vi "Crazy.vi"() -> ()   [LabVIEW 2014]
uses:
  <vilib>/Utility/inputDevices.llb/keyboardAcquire.vi
  <vilib>/Utility/inputDevices.llb/closeKeyboard.vi
panel:
  out "Å]YÄ²2":i32
  out "Å]XÄ²2":i32
  out "Å]Vy2":i32
  out "Å]Vx2":i32
  out "魔王2":bool
  out "Å]YÄ²1":i32
  out "Å]XÄ²1":i32
  out "Å]Vy1":i32
  out "Å]Vx1":i32
  out "魔王1":bool
  out "Vx 2":i32
  out "x觸及位置 2":i32
  out "X障礙 2":bool
  out "y觸及位置 2":i32
  out "Vy 2":i32
  out "Y障礙 2":bool
  out "Å]YÄ²":i32
  out "Å]XÄ²":i32
  out "Å]Vy":i64
  out "Å]Vx":i32
  out "魔王":bool
  out "終點":bool
  out "遊玩時間":i32
  out "X障礙":bool
  out "Y位置 2":i32
  out "x位置 2":i32
  out "X":dbl
  out "Y":dbl
  out "小精靈":bool
  out "x位置":i32
  out "Y位置":i32
  out "Y障礙":bool
  out "x觸及位置":i32
  out "y觸及位置":i32
  out "x-y":u32
  out "Vy":i32
  out "Vx":i32
  # "小精靈"
  # "500"
  # "障礙"
  # "400"
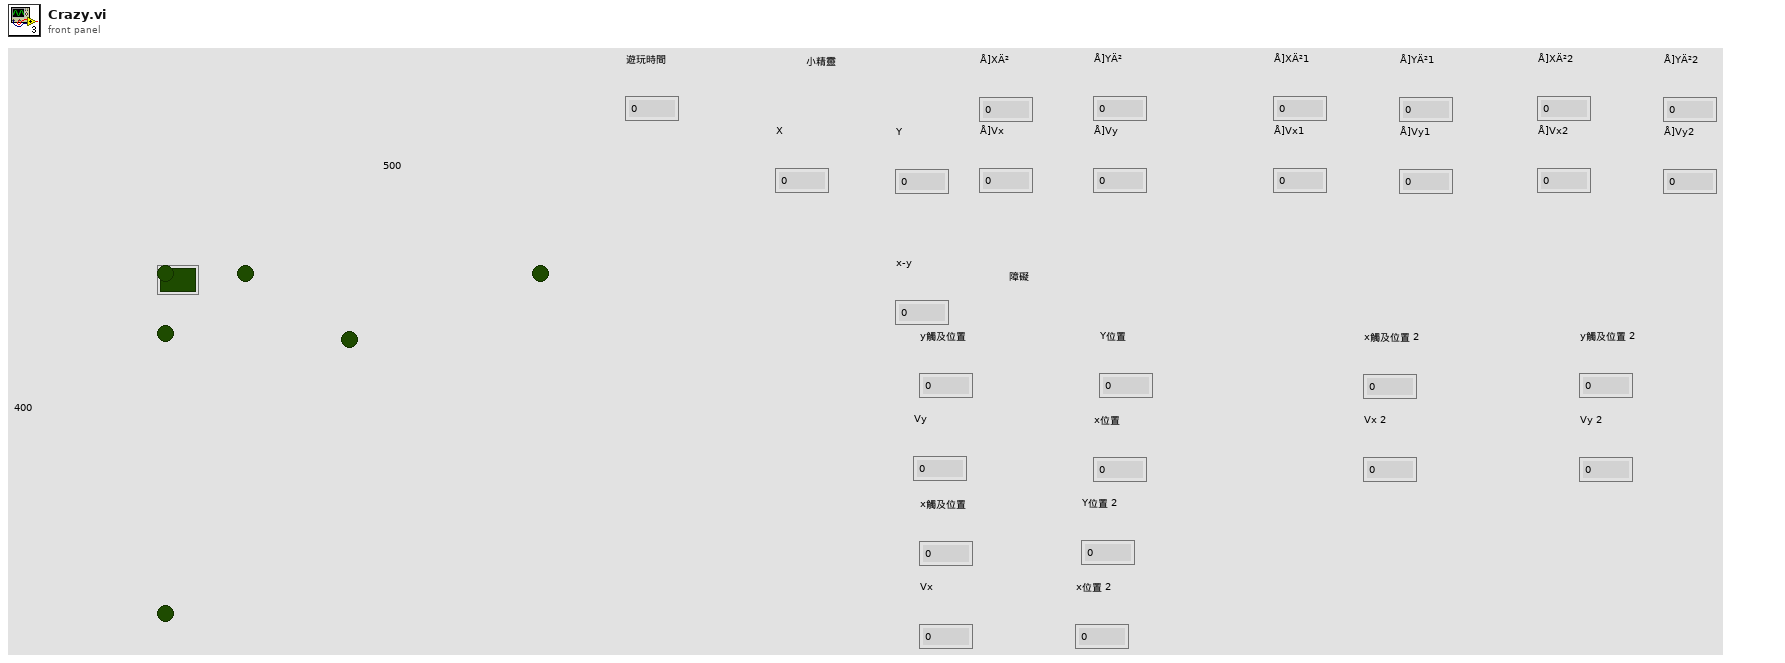
[diagram p1: front panel]
types:
  T1 = enum16{"0", "1", "2", "3", "4", "5", "6", "7", "8", "9", "A", "B", "C", "D", "E", "F", "G", "H", "I", "J", "K", "L", "M", "N", "O", "P", "Q", "R", "S", "T", "U", "V", "W", "X", "Y", "Z", "F1", "F2", "F3", "F4", "F5", "F6", "F7", "F8", "F9", "F10", "F11", "F12", "F13", "F14", "F15", "ADD", "BACK", "BACKSLASH", "CAPITAL", "COMMA", "DECIMAL", "DELETE", "DIVIDE", "DOWN", "END", "EQUALS", "ESCAPE", "GRAVE (`)", "HOME", "INSERT", "LBRACKET", "LCONTROL", "LEFT", "L ALT", "LSHIFT", "LWIN", "MINUS", "MULTIPLY", "NEXT", "NUMLOCK", "NUMPAD_0", "NUMPAD_1", "NUMPAD_2", "NUMPAD_3", "NUMPAD_4", "NUMPAD_5", "NUMPAD_6", "NUMPAD_7", "NUMPAD_8", "NUMPAD_9", "PAUSE", "PERIOD", "PRIOR (PG UP)", "RBRACKET", "RCONTROL", "RETURN", "RIGHT", "R ALT", "RSHIFT", "RWIN", "SCROLL", "SEMICOLON", "SLASH", "SPACE", "SUBTRACT", "TAB", "UP", "ENTER (num pad)", "' (quote)"}[]
  T2 = cluster{"keys pressed[0]":enum16{"0", "1", "2", "3", "4", "5", "6", "7", "8", "9", "A", "B", "C", "D", "E", "F", "G", "H", "I", "J", "K", "L", "M", "N", "O", "P", "Q", "R", "S", "T", "U", "V", "W", "X", "Y", "Z", "F1", "F2", "F3", "F4", "F5", "F6", "F7", "F8", "F9", "F10", "F11", "F12", "F13", "F14", "F15", "ADD", "BACK", "BACKSLASH", "CAPITAL", "COMMA", "DECIMAL", "DELETE", "DIVIDE", "DOWN", "END", "EQUALS", "ESCAPE", "GRAVE (`)", "HOME", "INSERT", "LBRACKET", "LCONTROL", "LEFT", "L ALT", "LSHIFT", "LWIN", "MINUS", "MULTIPLY", "NEXT", "NUMLOCK", "NUMPAD_0", "NUMPAD_1", "NUMPAD_2", "NUMPAD_3", "NUMPAD_4", "NUMPAD_5", "NUMPAD_6", "NUMPAD_7", "NUMPAD_8", "NUMPAD_9", "PAUSE", "PERIOD", "PRIOR (PG UP)", "RBRACKET", "RCONTROL", "RETURN", "RIGHT", "R ALT", "RSHIFT", "RWIN", "SCROLL", "SEMICOLON", "SLASH", "SPACE", "SUBTRACT", "TAB", "UP", "ENTER (num pad)", "' (quote)"}, "keys pressed[1]":enum16{"0", "1", "2", "3", "4", "5", "6", "7", "8", "9", "A", "B", "C", "D", "E", "F", "G", "H", "I", "J", "K", "L", "M", "N", "O", "P", "Q", "R", "S", "T", "U", "V", "W", "X", "Y", "Z", "F1", "F2", "F3", "F4", "F5", "F6", "F7", "F8", "F9", "F10", "F11", "F12", "F13", "F14", "F15", "ADD", "BACK", "BACKSLASH", "CAPITAL", "COMMA", "DECIMAL", "DELETE", "DIVIDE", "DOWN", "END", "EQUALS", "ESCAPE", "GRAVE (`)", "HOME", "INSERT", "LBRACKET", "LCONTROL", "LEFT", "L ALT", "LSHIFT", "LWIN", "MINUS", "MULTIPLY", "NEXT", "NUMLOCK", "NUMPAD_0", "NUMPAD_1", "NUMPAD_2", "NUMPAD_3", "NUMPAD_4", "NUMPAD_5", "NUMPAD_6", "NUMPAD_7", "NUMPAD_8", "NUMPAD_9", "PAUSE", "PERIOD", "PRIOR (PG UP)", "RBRACKET", "RCONTROL", "RETURN", "RIGHT", "R ALT", "RSHIFT", "RWIN", "SCROLL", "SEMICOLON", "SLASH", "SPACE", "SUBTRACT", "TAB", "UP", "ENTER (num pad)", "' (quote)"}, "keys pressed[2]":enum16{"0", "1", "2", "3", "4", "5", "6", "7", "8", "9", "A", "B", "C", "D", "E", "F", "G", "H", "I", "J", "K", "L", "M", "N", "O", "P", "Q", "R", "S", "T", "U", "V", "W", "X", "Y", "Z", "F1", "F2", "F3", "F4", "F5", "F6", "F7", "F8", "F9", "F10", "F11", "F12", "F13", "F14", "F15", "ADD", "BACK", "BACKSLASH", "CAPITAL", "COMMA", "DECIMAL", "DELETE", "DIVIDE", "DOWN", "END", "EQUALS", "ESCAPE", "GRAVE (`)", "HOME", "INSERT", "LBRACKET", "LCONTROL", "LEFT", "L ALT", "LSHIFT", "LWIN", "MINUS", "MULTIPLY", "NEXT", "NUMLOCK", "NUMPAD_0", "NUMPAD_1", "NUMPAD_2", "NUMPAD_3", "NUMPAD_4", "NUMPAD_5", "NUMPAD_6", "NUMPAD_7", "NUMPAD_8", "NUMPAD_9", "PAUSE", "PERIOD", "PRIOR (PG UP)", "RBRACKET", "RCONTROL", "RETURN", "RIGHT", "R ALT", "RSHIFT", "RWIN", "SCROLL", "SEMICOLON", "SLASH", "SPACE", "SUBTRACT", "TAB", "UP", "ENTER (num pad)", "' (quote)"}, "keys pressed[3]":enum16{"0", "1", "2", "3", "4", "5", "6", "7", "8", "9", "A", "B", "C", "D", "E", "F", "G", "H", "I", "J", "K", "L", "M", "N", "O", "P", "Q", "R", "S", "T", "U", "V", "W", "X", "Y", "Z", "F1", "F2", "F3", "F4", "F5", "F6", "F7", "F8", "F9", "F10", "F11", "F12", "F13", "F14", "F15", "ADD", "BACK", "BACKSLASH", "CAPITAL", "COMMA", "DECIMAL", "DELETE", "DIVIDE", "DOWN", "END", "EQUALS", "ESCAPE", "GRAVE (`)", "HOME", "INSERT", "LBRACKET", "LCONTROL", "LEFT", "L ALT", "LSHIFT", "LWIN", "MINUS", "MULTIPLY", "NEXT", "NUMLOCK", "NUMPAD_0", "NUMPAD_1", "NUMPAD_2", "NUMPAD_3", "NUMPAD_4", "NUMPAD_5", "NUMPAD_6", "NUMPAD_7", "NUMPAD_8", "NUMPAD_9", "PAUSE", "PERIOD", "PRIOR (PG UP)", "RBRACKET", "RCONTROL", "RETURN", "RIGHT", "R ALT", "RSHIFT", "RWIN", "SCROLL", "SEMICOLON", "SLASH", "SPACE", "SUBTRACT", "TAB", "UP", "ENTER (num pad)", "' (quote)"}, "keys pressed[4]":enum16{"0", "1", "2", "3", "4", "5", "6", "7", "8", "9", "A", "B", "C", "D", "E", "F", "G", "H", "I", "J", "K", "L", "M", "N", "O", "P", "Q", "R", "S", "T", "U", "V", "W", "X", "Y", "Z", "F1", "F2", "F3", "F4", "F5", "F6", "F7", "F8", "F9", "F10", "F11", "F12", "F13", "F14", "F15", "ADD", "BACK", "BACKSLASH", "CAPITAL", "COMMA", "DECIMAL", "DELETE", "DIVIDE", "DOWN", "END", "EQUALS", "ESCAPE", "GRAVE (`)", "HOME", "INSERT", "LBRACKET", "LCONTROL", "LEFT", "L ALT", "LSHIFT", "LWIN", "MINUS", "MULTIPLY", "NEXT", "NUMLOCK", "NUMPAD_0", "NUMPAD_1", "NUMPAD_2", "NUMPAD_3", "NUMPAD_4", "NUMPAD_5", "NUMPAD_6", "NUMPAD_7", "NUMPAD_8", "NUMPAD_9", "PAUSE", "PERIOD", "PRIOR (PG UP)", "RBRACKET", "RCONTROL", "RETURN", "RIGHT", "R ALT", "RSHIFT", "RWIN", "SCROLL", "SEMICOLON", "SLASH", "SPACE", "SUBTRACT", "TAB", "UP", "ENTER (num pad)", "' (quote)"}, "keys pressed[5]":enum16{"0", "1", "2", "3", "4", "5", "6", "7", "8", "9", "A", "B", "C", "D", "E", "F", "G", "H", "I", "J", "K", "L", "M", "N", "O", "P", "Q", "R", "S", "T", "U", "V", "W", "X", "Y", "Z", "F1", "F2", "F3", "F4", "F5", "F6", "F7", "F8", "F9", "F10", "F11", "F12", "F13", "F14", "F15", "ADD", "BACK", "BACKSLASH", "CAPITAL", "COMMA", "DECIMAL", "DELETE", "DIVIDE", "DOWN", "END", "EQUALS", "ESCAPE", "GRAVE (`)", "HOME", "INSERT", "LBRACKET", "LCONTROL", "LEFT", "L ALT", "LSHIFT", "LWIN", "MINUS", "MULTIPLY", "NEXT", "NUMLOCK", "NUMPAD_0", "NUMPAD_1", "NUMPAD_2", "NUMPAD_3", "NUMPAD_4", "NUMPAD_5", "NUMPAD_6", "NUMPAD_7", "NUMPAD_8", "NUMPAD_9", "PAUSE", "PERIOD", "PRIOR (PG UP)", "RBRACKET", "RCONTROL", "RETURN", "RIGHT", "R ALT", "RSHIFT", "RWIN", "SCROLL", "SEMICOLON", "SLASH", "SPACE", "SUBTRACT", "TAB", "UP", "ENTER (num pad)", "' (quote)"}, "keys pressed[6]":enum16{"0", "1", "2", "3", "4", "5", "6", "7", "8", "9", "A", "B", "C", "D", "E", "F", "G", "H", "I", "J", "K", "L", "M", "N", "O", "P", "Q", "R", "S", "T", "U", "V", "W", "X", "Y", "Z", "F1", "F2", "F3", "F4", "F5", "F6", "F7", "F8", "F9", "F10", "F11", "F12", "F13", "F14", "F15", "ADD", "BACK", "BACKSLASH", "CAPITAL", "COMMA", "DECIMAL", "DELETE", "DIVIDE", "DOWN", "END", "EQUALS", "ESCAPE", "GRAVE (`)", "HOME", "INSERT", "LBRACKET", "LCONTROL", "LEFT", "L ALT", "LSHIFT", "LWIN", "MINUS", "MULTIPLY", "NEXT", "NUMLOCK", "NUMPAD_0", "NUMPAD_1", "NUMPAD_2", "NUMPAD_3", "NUMPAD_4", "NUMPAD_5", "NUMPAD_6", "NUMPAD_7", "NUMPAD_8", "NUMPAD_9", "PAUSE", "PERIOD", "PRIOR (PG UP)", "RBRACKET", "RCONTROL", "RETURN", "RIGHT", "R ALT", "RSHIFT", "RWIN", "SCROLL", "SEMICOLON", "SLASH", "SPACE", "SUBTRACT", "TAB", "UP", "ENTER (num pad)", "' (quote)"}, "keys pressed[7]":enum16{"0", "1", "2", "3", "4", "5", "6", "7", "8", "9", "A", "B", "C", "D", "E", "F", "G", "H", "I", "J", "K", "L", "M", "N", "O", "P", "Q", "R", "S", "T", "U", "V", "W", "X", "Y", "Z", "F1", "F2", "F3", "F4", "F5", "F6", "F7", "F8", "F9", "F10", "F11", "F12", "F13", "F14", "F15", "ADD", "BACK", "BACKSLASH", "CAPITAL", "COMMA", "DECIMAL", "DELETE", "DIVIDE", "DOWN", "END", "EQUALS", "ESCAPE", "GRAVE (`)", "HOME", "INSERT", "LBRACKET", "LCONTROL", "LEFT", "L ALT", "LSHIFT", "LWIN", "MINUS", "MULTIPLY", "NEXT", "NUMLOCK", "NUMPAD_0", "NUMPAD_1", "NUMPAD_2", "NUMPAD_3", "NUMPAD_4", "NUMPAD_5", "NUMPAD_6", "NUMPAD_7", "NUMPAD_8", "NUMPAD_9", "PAUSE", "PERIOD", "PRIOR (PG UP)", "RBRACKET", "RCONTROL", "RETURN", "RIGHT", "R ALT", "RSHIFT", "RWIN", "SCROLL", "SEMICOLON", "SLASH", "SPACE", "SUBTRACT", "TAB", "UP", "ENTER (num pad)", "' (quote)"}, "keys pressed[8]":enum16{"0", "1", "2", "3", "4", "5", "6", "7", "8", "9", "A", "B", "C", "D", "E", "F", "G", "H", "I", "J", "K", "L", "M", "N", "O", "P", "Q", "R", "S", "T", "U", "V", "W", "X", "Y", "Z", "F1", "F2", "F3", "F4", "F5", "F6", "F7", "F8", "F9", "F10", "F11", "F12", "F13", "F14", "F15", "ADD", "BACK", "BACKSLASH", "CAPITAL", "COMMA", "DECIMAL", "DELETE", "DIVIDE", "DOWN", "END", "EQUALS", "ESCAPE", "GRAVE (`)", "HOME", "INSERT", "LBRACKET", "LCONTROL", "LEFT", "L ALT", "LSHIFT", "LWIN", "MINUS", "MULTIPLY", "NEXT", "NUMLOCK", "NUMPAD_0", "NUMPAD_1", "NUMPAD_2", "NUMPAD_3", "NUMPAD_4", "NUMPAD_5", "NUMPAD_6", "NUMPAD_7", "NUMPAD_8", "NUMPAD_9", "PAUSE", "PERIOD", "PRIOR (PG UP)", "RBRACKET", "RCONTROL", "RETURN", "RIGHT", "R ALT", "RSHIFT", "RWIN", "SCROLL", "SEMICOLON", "SLASH", "SPACE", "SUBTRACT", "TAB", "UP", "ENTER (num pad)", "' (quote)"}}
  T3 = enum16{"0", "1", "2", "3", "4", "5", "6", "7", "8", "9", "A", "B", "C", "D", "E", "F", "G", "H", "I", "J", "K", "L", "M", "N", "O", "P", "Q", "R", "S", "T", "U", "V", "W", "X", "Y", "Z", "F1", "F2", "F3", "F4", "F5", "F6", "F7", "F8", "F9", "F10", "F11", "F12", "F13", "F14", "F15", "ADD", "BACK", "BACKSLASH", "CAPITAL", "COMMA", "DECIMAL", "DELETE", "DIVIDE", "DOWN", "END", "EQUALS", "ESCAPE", "GRAVE (`)", "HOME", "INSERT", "LBRACKET", "LCONTROL", "LEFT", "L ALT", "LSHIFT", "LWIN", "MINUS", "MULTIPLY", "NEXT", "NUMLOCK", "NUMPAD_0", "NUMPAD_1", "NUMPAD_2", "NUMPAD_3", "NUMPAD_4", "NUMPAD_5", "NUMPAD_6", "NUMPAD_7", "NUMPAD_8", "NUMPAD_9", "PAUSE", "PERIOD", "PRIOR (PG UP)", "RBRACKET", "RCONTROL", "RETURN", "RIGHT", "R ALT", "RSHIFT", "RWIN", "SCROLL", "SEMICOLON", "SLASH", "SPACE", "SUBTRACT", "TAB", "UP", "ENTER (num pad)", "' (quote)"}
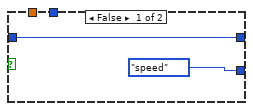
[diagram p3: hidden frame]
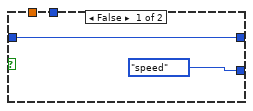
[diagram p5: hidden frame]
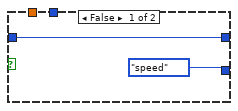
[diagram p7: hidden frame]
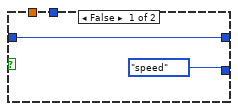
[diagram p9: hidden frame]
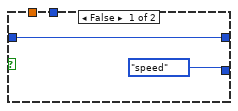
[diagram p11: hidden frame]
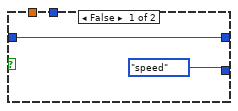
[diagram p17: hidden frame]
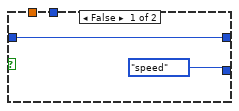
[diagram p19: hidden frame]
diagram:
  n1 = flat-sequence {
    tunnel: [w107] -> w32
    tunnel: [w106] -> w30
    tunnel: [w99] -> w18
    tunnel: [w98] -> w17
    tunnel: [w91] -> w5
    tunnel: [w589] -> w33
    tunnel: w32 -> [w589]
    tunnel: [w588] -> w31
    tunnel: w30 -> [w588]
    tunnel: w18 -> [w567]
    tunnel: w17 -> [w568]
    tunnel: [w568] -> w16
    tunnel: [w567] -> w15
    tunnel: [w566] -> w6
    tunnel: w5 -> [w566]
    tunnel: w33 -> [w633]
    tunnel: w31 -> [w632]
    tunnel: [w623] -> w27
    tunnel: [w622] -> w25
    tunnel: [w621] -> w23
    tunnel: [w620] -> w21
    tunnel: [w619] -> w19
    tunnel: w16 -> [w612]
    tunnel: w15 -> [w611]
    tunnel: [w610] -> w14
    tunnel: [w609] -> w13
    tunnel: [w608] -> w10
    tunnel: [w607] -> w9
    tunnel: w6 -> [w606]
    tunnel: [w605] -> w3
    tunnel: [w598] -> w1
    tunnel: [w1256] -> w28
    tunnel: w27 -> [w1256]
    tunnel: [w1255] -> w26
    tunnel: w25 -> [w1255]
    tunnel: [w1254] -> w24
    tunnel: w23 -> [w1254]
    tunnel: [w1253] -> w22
    tunnel: w21 -> [w1253]
    tunnel: [w1252] -> w20
    tunnel: w19 -> [w1252]
    tunnel: w14 -> [w1237]
    tunnel: w13 -> [w1236]
    tunnel: [w1237] -> w12
    tunnel: [w1236] -> w11
    tunnel: w10 -> [w1235]
    tunnel: w9 -> [w1234]
    tunnel: [w1235] -> w8
    tunnel: [w1234] -> w7
    tunnel: [w1225] -> w4
    tunnel: w3 -> [w1225]
    tunnel: [w1224] -> w2
    tunnel: w1 -> [w1224]
    tunnel: w28 -> [w1300]
    tunnel: w26 -> [w1299]
    tunnel: w24 -> [w1298]
    tunnel: w22 -> [w1297]
    tunnel: w20 -> [w1296]
    tunnel: w12 -> [w1278]
    tunnel: w11 -> [w1277]
    tunnel: w8 -> [w1276]
    tunnel: w7 -> [w1275]
    tunnel: w4 -> [w1268]
    tunnel: w2 -> [w1267]
    frame #0 {
      w38 = 0 ("Å]XÄ²1")
      # "下:小精靈控制"
      # "上:障礙控制"
      n2 = Random Number (0-1)() -> (number: 0 to 1=w80:dbl)
      n3 = Random Number (0-1)() -> (number: 0 to 1=w47:dbl)
      n4 = Random Number (0-1)() -> (number: 0 to 1=w85:dbl)
      n5 = Random Number (0-1)() -> (number: 0 to 1=w41:dbl)
      n6 = Multiply(x=200.0, y=w80) -> (x*y=w78:dbl)
      n7 = Random Number (0-1)() -> (number: 0 to 1=w54:dbl)
      n8 = property on="Y障礙 2" class="Bool (strict)"("Left"=300 ("Position:Left"), "Top"=1 ("Position:Top")) -> ()  [unwired: 2 in, 2 out]
      n9 = Random Number (0-1)() -> (number: 0 to 1=w62:dbl)
      n10 = property on="Y障礙" class="Bool (strict)"("Left"=200 ("Position:Left"), "Top"=1 ("Position:Top")) -> ()  [unwired: 2 in, 2 out]
      n11 = property on="魔王" class="Bool (strict)"("Left"=-500 ("Position:Left"), "Top"=0 ("Position:Top")) -> ()  [unwired: 2 in, 2 out]
      n12 = Add(x=100.0 ("Vy"), y=w78) -> (x+y=→"Vy":dbl)
      n13 = Multiply(x=200.0, y=w54) -> (x*y=w52:dbl)
      n14 = Multiply(x=200.0, y=w47) -> (x*y=w45:dbl)
      n15 = Add(x=300.0 ("y"), y=w45) -> (x+y=→"Å]Vx1":dbl)
      n16 = Multiply(x=200.0, y=w85) -> (x*y=w83:dbl)
      n17 = Add(x=100.0 ("y"), y=w83) -> (x+y=→"Vx":dbl)
      n18 = Multiply(x=200.0, y=w41) -> (x*y=w43:dbl)
      n19 = Add(x=300.0 ("y"), y=w43) -> (x+y=→"Å]Vy1":dbl)
      n20 = Add(x=100.0 ("Vy"), y=w52) -> (x+y=→"Vy 2":dbl)
      n21 = Multiply(x=200.0, y=w62) -> (x*y=w60:dbl)
      n22 = Add(x=100.0 ("y"), y=w60) -> (x+y=→"Vx 2":dbl)
      n23 = property on="小精靈" class="Bool (strict)"("Left"=0 ("Position:Left"), "Top"=100 ("Position:Top")) -> ()  [unwired: 2 in, 2 out]
      n24 = property on="終點" class="Bool (strict)"("Left"=477 ("Position:Left"), "Top"=374 ("Position:Top")) -> ()  [unwired: 2 in, 2 out]
      n25 = property on="X障礙" class="Bool (strict)"("Left"=1 ("Position:Left"), "Top"=200 ("Position:Top")) -> ()  [unwired: 2 in, 2 out]
      n26 = property on="魔王1" class="Bool (strict)"("Left"=-500 ("Position:Left"), "Top"=0 ("Position:Top")) -> ()  [unwired: 2 in, 2 out]
      n27 = property on="魔王2" class="Bool (strict)"("Left"=-500 ("Position:Left"), "Top"=5 ("Position:Top")) -> ()  [unwired: 2 in, 2 out]
      n28 = property on="X障礙 2" class="Bool (strict)"("Left"=1 ("Position:Left"), "Top"=270 ("Position:Top")) -> ()  [unwired: 2 in, 2 out]
      "y觸及位置" <- 0.0 ("x*y")
      "x觸及位置" <- 0.0 ("x*y")
      "小精靈" <- TRUE
      "X" <- 0.0 ("Numeric")
      "Y" <- 100.0 ("Y")
      "遊玩時間" <- 0 ("Numeric")
      "x觸及位置 2" <- 0.0 ("x*y")
      "y觸及位置 2" <- 0.0 ("x*y")
      "Å]XÄ²1" <- w38
      "Å]YÄ²1" <- w38
    }
    frame #1 {
      w92 = 0 ("Top")
      w95 = 0 ("Top")
      w102 = 0 ("Left")
      w103 = 0 ("Left")
      w108 = 0
      w109 = 0
      n29 = call <vilib>:"Intialize Keyboard.vi"() -> ("error out"=w113:errorcluster, "device ID"=w115:refnum<k1>)  [unwired: 10 in]
      n30 = Tick Count (ms)() -> (millisecond timer value=w116:u32)
      n31 = Tick Count (ms)() -> (millisecond timer value=w111:u32)
      n32 = Tick Count (ms)() -> (millisecond timer value=w94:u32)
      n33 = Tick Count (ms)() -> (millisecond timer value=w101:u32)
      n34 = Tick Count (ms)() -> (millisecond timer value=w105:u32)
      n35 = Tick Count (ms)() -> (millisecond timer value=w97:u32)
      n36 = while {
        shift-right: [w257] -> _
        shift-left: enum16{"speed"}."speed" ("Enum") -> [w259]
        shift-right: [w258] -> _
        shift-left: w116 -> [w260]
        tunnel: w115 -> [w256]
        tunnel: [w223] -> w114
        tunnel: w113 -> [w255]
        tunnel: [w222] -> w112
        shift-right: [w251] -> _
        shift-left: w111 -> [w252]
        shift-right: [w250] -> _
        shift-left: enum16{"speed"}."speed" ("Enum") -> [w249]
        shift-right: [w246] -> _
        shift-left: w109 -> [w244]
        shift-left: w109 -> [w243]
        shift-right: [w245] -> _
        shift-left: w108 -> [w242]
        shift-left: w108 -> [w241]
        tunnel: [w204] -> w107
        tunnel: [w203] -> w106
        shift-right: [w193] -> _
        shift-left: w105 -> [w195]
        shift-right: [w194] -> _
        shift-left: enum16{"speed"}."speed" ("Enum") -> [w196]
        shift-right: [w192] -> _
        shift-left: w103 -> [w191]
        shift-left: w103 -> [w190]
        shift-right: [w189] -> _
        shift-left: w102 -> [w188]
        shift-left: w102 -> [w187]
        shift-right: [w184] -> _
        shift-left: w101 -> [w186]
        shift-right: [w183] -> _
        shift-left: enum16{"speed"}."speed" ("Enum") -> [w185]
        tunnel: [w149] -> w99
        tunnel: [w150] -> w98
        shift-right: [w146] -> _
        shift-left: w97 -> [w148]
        shift-right: [w145] -> _
        shift-left: enum16{"speed"}."speed" ("Enum") -> [w147]
        shift-right: [w144] -> _
        shift-left: w95 -> [w143]
        shift-left: w95 -> [w142]
        shift-right: [w139] -> _
        shift-left: w94 -> [w141]
        shift-right: [w138] -> _
        shift-left: enum16{"speed"}."speed" ("Enum") -> [w140]
        shift-right: [w137] -> _
        shift-left: w92 -> [w136]
        shift-left: w92 -> [w135]
        tunnel: [w118] -> w91
        stop <- w202 stop-if-true
        n37 = local read "遊玩時間"() -> (w201:i32)
        n38 = property on="小精靈" class="Bool (strict)"() -> ("Left"=w248:i32)  [unwired: 2 in, 2 out]
        n39 = case shown="\"speed\"" w249 {
          tunnel: w252 -> [w476]
          tunnel: [w475] -> w251
          tunnel: [w474] -> w250
          tunnel: w244 -> [w464]
          tunnel: w243 -> [w463]
          tunnel: w244 -> [w458]
          tunnel: w243 -> [w457]
          tunnel: [w452] -> w246
          tunnel: w244 -> [_]
          tunnel: w243 -> [_]
          frame "speed" {
            n40 = Tick Count (ms)() -> (millisecond timer value=w485:u32)
            n41 = Greater?(x=w464, y=500.0) -> (0:w460:bool)
            n42 = Greater?(x=w463, y=500.0) -> (0:w459:bool)
            n43 = Less?(x=w458, y=0.0) -> (x < y?=w454:bool)
            n44 = Less?(x=w457, y=0.0) -> (x < y?=w453:bool)
            n45 = property on="X障礙" class="Bool (strict)"() -> ("Left"=w477:i32)  [unwired: 2 in, 2 out]
            n46 = property on="X障礙" class="Bool (strict)"() -> ("Left"=w471:i32)  [unwired: 2 in, 2 out]
            n47 = Less?(x=w471, y=0) -> (x < y?=w469:bool)
            n48 = Greater?(x=w477, y=500) -> (0:w468:bool)
            n49 = And(x=w460, y=w459) -> (x .and. y?=w451:bool)
            n50 = And(x=w454, y=w453) -> (x .and. y?=w450:bool)
            n51 = Subtract(x=w485, y=w476) -> (x-y=w484:u32)
            n52 = Or(x=w468, y=w469) -> (x .or. y?=w467:bool)
            n53 = To Double Precision Float(number=w484) -> (double precision float=w483:dbl)
            n54 = Compound Arithmetic op=OR(w451, w450) -> (w449:bool)
            n55 = local read "Vx"() -> (w473:i32)
            n56 = local read "x觸及位置"() -> (w479:i32)
            n57 = Divide(x=w483, y=1000.0) -> (x/y=w481:dbl)
            n58 = case shown="True" w449 {
              frame False {
              }
              frame True {
                w486 = 200 ("x觸及位置")
                n59 = local write "x觸及位置"(w486) -> ()
                n60 = Wait (ms)(milliseconds to wait=u32 100) -> ()  [unwired: 1 out]
                n61 = property on="X障礙" class="Bool (strict)"("Left"=w486) -> ()  [unwired: 2 in, 2 out]
              }
            }
            n62 = Multiply(x=w481, y=w473) -> (x*y=w480:dbl)
            n63 = Add(x=w480, y=w479) -> (x+y=w465:dbl)
            n64 = case shown="True" w467 {
              tunnel: [enum16{"speed"}."speed" ("Enum") enum16{"speed"}."speed" ("Enum")] -> w474
              tunnel: [w488 w495] -> w475
              tunnel: w476 -> [w488 _]
              tunnel: w465 -> [_ w492]
              tunnel: w473 -> [_ w494]
              frame False {
              }
              frame True {
                n65 = local write "x觸及位置"(w492) -> ()
                n66 = Multiply(x=w494, y=-1.0) -> (x*y=w491:dbl)
                n67 = Wait (ms)(milliseconds to wait=u32 25) -> ()  [unwired: 1 out]
                n68 = Tick Count (ms)() -> (millisecond timer value=w495:u32)
                n69 = local write "Vx"(w491) -> ()
              }
            }
            n70 = property on="X障礙" class="Bool (strict)"("Left"=w465) -> ()  [unwired: 2 in, 2 out]
            n71 = property on="X障礙" class="Bool (strict)"() -> ("Top"=→"Y位置 2":i32, "Left"=w452:i32)  [unwired: 2 in, 2 out]
            "x位置 2" <- w452
            n72 = Wait (ms)(milliseconds to wait=u32 10) -> ()  [unwired: 1 out]
          }
        }
        n73 = case shown="\"speed\"" w196 {
          tunnel: w195 -> [w428]
          tunnel: [w427] -> w193
          tunnel: [w426] -> w194
          tunnel: w191 -> [w417]
          tunnel: w190 -> [w416]
          tunnel: w191 -> [w411]
          tunnel: w190 -> [w410]
          tunnel: [w402] -> w192
          frame "speed" {
            n74 = Tick Count (ms)() -> (millisecond timer value=w437:u32)
            n75 = Greater?(x=w417, y=500.0) -> (0:w413:bool)
            n76 = Greater?(x=w416, y=500.0) -> (0:w412:bool)
            n77 = Less?(x=w411, y=0.0) -> (x < y?=w407:bool)
            n78 = Less?(x=w410, y=0.0) -> (x < y?=w406:bool)
            n79 = property on="X障礙 2" class="Bool (strict)"() -> ("Left"=w429:i32)  [unwired: 2 in, 2 out]
            n80 = property on="X障礙 2" class="Bool (strict)"() -> ("Left"=w423:i32)  [unwired: 2 in, 2 out]
            n81 = Less?(x=w423, y=0) -> (x < y?=w421:bool)
            n82 = Greater?(x=w429, y=500) -> (0:w420:bool)
            n83 = And(x=w413, y=w412) -> (x .and. y?=w405:bool)
            n84 = And(x=w407, y=w406) -> (x .and. y?=w404:bool)
            n85 = Subtract(x=w437, y=w428) -> (x-y=w436:u32)
            n86 = Or(x=w420, y=w421) -> (x .or. y?=w419:bool)
            n87 = To Double Precision Float(number=w436) -> (double precision float=w435:dbl)
            n88 = Compound Arithmetic op=OR(w405, w404) -> (w403:bool)
            n89 = local read "Vx 2"() -> (w425:i32)
            n90 = local read "x觸及位置 2"() -> (w431:i32)
            n91 = Divide(x=w435, y=1000.0) -> (x/y=w433:dbl)
            n92 = case shown="True" w403 {
              frame False {
              }
              frame True {
                w438 = 200 ("x觸及位置")
                n93 = local write "x觸及位置 2"(w438) -> ()
                n94 = property on="X障礙 2" class="Bool (strict)"("Left"=w438) -> ()  [unwired: 2 in, 2 out]
                n95 = Wait (ms)(milliseconds to wait=u32 100) -> ()  [unwired: 1 out]
              }
            }
            n96 = Multiply(x=w433, y=w425) -> (x*y=w432:dbl)
            n97 = Add(x=w432, y=w431) -> (x+y=w418:dbl)
            n98 = case shown="True" w419 {
              tunnel: [enum16{"speed"}."speed" ("Enum") enum16{"speed"}."speed" ("Enum")] -> w426
              tunnel: [w440 w447] -> w427
              tunnel: w428 -> [w440 _]
              tunnel: w418 -> [_ w444]
              tunnel: w425 -> [_ w446]
              frame False {
              }
              frame True {
                n99 = local write "x觸及位置 2"(w444) -> ()
                n100 = Multiply(x=w446, y=-1.0) -> (x*y=w443:dbl)
                n101 = Wait (ms)(milliseconds to wait=u32 25) -> ()  [unwired: 1 out]
                n102 = local write "Vx 2"(w443) -> ()
                n103 = Tick Count (ms)() -> (millisecond timer value=w447:u32)
              }
            }
            n104 = property on="X障礙 2" class="Bool (strict)"("Left"=w418) -> ()  [unwired: 2 in, 2 out]
            n105 = property on="X障礙 2" class="Bool (strict)"() -> ("Left"=w402:i32)  [unwired: 2 in, 2 out]
            n106 = Wait (ms)(milliseconds to wait=u32 10) -> ()  [unwired: 1 out]
          }
        }
        n107 = local read "遊玩時間"() -> (w199:i32)
        n108 = case shown="\"speed\"" w185 {
          tunnel: w186 -> [w381]
          tunnel: [w380] -> w184
          tunnel: [w379] -> w183
          tunnel: w188 -> [w370]
          tunnel: w187 -> [w369]
          tunnel: w188 -> [w364]
          tunnel: w187 -> [w363]
          tunnel: [w355] -> w189
          frame "speed" {
            n109 = Tick Count (ms)() -> (millisecond timer value=w390:u32)
            n110 = Greater?(x=w370, y=400.0) -> (0:w366:bool)
            n111 = Greater?(x=w369, y=400.0) -> (0:w365:bool)
            n112 = Less?(x=w364, y=0.0) -> (x < y?=w360:bool)
            n113 = Less?(x=w363, y=0.0) -> (x < y?=w359:bool)
            n114 = property on="Y障礙 2" class="Bool (strict)"() -> ("Top"=w382:i32)  [unwired: 2 in, 2 out]
            n115 = property on="Y障礙 2" class="Bool (strict)"() -> ("Top"=w376:i32)  [unwired: 2 in, 2 out]
            n116 = Less?(x=w376, y=0) -> (x < y?=w374:bool)
            n117 = Greater?(x=w382, y=400) -> (0:w373:bool)
            n118 = And(x=w366, y=w365) -> (x .and. y?=w358:bool)
            n119 = And(x=w360, y=w359) -> (x .and. y?=w357:bool)
            n120 = Subtract(x=w390, y=w381) -> (x-y=w389:u32)
            n121 = Or(x=w373, y=w374) -> (x .or. y?=w372:bool)
            n122 = To Double Precision Float(number=w389) -> (double precision float=w388:dbl)
            n123 = Compound Arithmetic op=OR(w358, w357) -> (w356:bool)
            n124 = local read "Vy 2"() -> (w378:i32)
            n125 = local read "y觸及位置 2"() -> (w384:i32)
            n126 = Divide(x=w388, y=1000.0) -> (x/y=w386:dbl)
            n127 = case shown="True" w356 {
              frame False {
              }
              frame True {
                w391 = 200 ("x觸及位置")
                n128 = local write "y觸及位置 2"(w391) -> ()
                n129 = property on="Y障礙 2" class="Bool (strict)"("Top"=w391) -> ()  [unwired: 2 in, 2 out]
                n130 = Wait (ms)(milliseconds to wait=u32 100) -> ()  [unwired: 1 out]
              }
            }
            n131 = Multiply(x=w386, y=w378) -> (x*y=w385:dbl)
            n132 = Add(x=w385, y=w384) -> (x+y=w371:dbl)
            n133 = case shown="True" w372 {
              tunnel: [enum16{"speed"}."speed" ("Enum") enum16{"speed"}."speed" ("Enum")] -> w379
              tunnel: [w393 w400] -> w380
              tunnel: w381 -> [w393 _]
              tunnel: w371 -> [_ w397]
              tunnel: w378 -> [_ w399]
              frame False {
              }
              frame True {
                n134 = local write "y觸及位置 2"(w397) -> ()
                n135 = Multiply(x=w399, y=-1.0) -> (x*y=w396:dbl)
                n136 = Wait (ms)(milliseconds to wait=u32 25) -> ()  [unwired: 1 out]
                n137 = local write "Vy 2"(w396) -> ()
                n138 = Tick Count (ms)() -> (millisecond timer value=w400:u32)
              }
            }
            n139 = property on="Y障礙 2" class="Bool (strict)"("Top"=w371) -> ()  [unwired: 2 in, 2 out]
            n140 = property on="Y障礙 2" class="Bool (strict)"() -> ("Top"=w355:i32)  [unwired: 2 in, 2 out]
            n141 = Wait (ms)(milliseconds to wait=u32 10) -> ()  [unwired: 1 out]
          }
        }
        n142 = case shown="\"speed\"" w147 {
          tunnel: w148 -> [w334]
          tunnel: [w332] -> w146
          tunnel: [w331] -> w145
          tunnel: [w315] -> w144
          tunnel: w143 -> [w314]
          tunnel: w143 -> [w313]
          tunnel: w142 -> [w312]
          tunnel: w142 -> [w311]
          frame "speed" {
            n143 = Tick Count (ms)() -> (millisecond timer value=w343:u32)
            n144 = property on="魔王1" class="Bool (strict)"() -> ("Top"=w335:i32)  [unwired: 2 in, 2 out]
            n145 = property on="魔王1" class="Bool (strict)"() -> ("Top"=w329:i32)  [unwired: 2 in, 2 out]
            n146 = Less?(x=w329, y=0) -> (x < y?=w327:bool)
            n147 = Greater?(x=w314, y=400.0) -> (0:w309:bool)
            n148 = Greater?(x=w312, y=400.0) -> (0:w318:bool)
            n149 = Less?(x=w313, y=0.0) -> (x < y?=w321:bool)
            n150 = Less?(x=w311, y=0.0) -> (x < y?=w322:bool)
            n151 = Greater?(x=w335, y=400) -> (0:w326:bool)
            n152 = Subtract(x=w343, y=w334) -> (x-y=w342:u32)
            n153 = Or(x=w326, y=w327) -> (x .or. y?=w325:bool)
            n154 = To Double Precision Float(number=w342) -> (double precision float=w341:dbl)
            n155 = And(x=w309, y=w318) -> (x .and. y?=w323:bool)
            n156 = And(x=w321, y=w322) -> (x .and. y?=w324:bool)
            n157 = local read "Å]Vy1"() -> (w330:i32)
            n158 = Or(x=w323, y=w324) -> (x .or. y?=w310:bool)
            n159 = Divide(x=w341, y=1000.0) -> (x/y=w339:dbl)
            n160 = local read "Å]YÄ²1"() -> (w337:i32)
            n161 = case shown="True" w310 {
              frame False {
              }
              frame True {
                w344 = 200 ("x觸及位置")
                n162 = local write "Å]YÄ²1"(w344) -> ()
                n163 = Wait (ms)(milliseconds to wait=u32 100) -> ()  [unwired: 1 out]
                n164 = property on="魔王1" class="Bool (strict)"("Top"=w344) -> ()  [unwired: 2 in, 2 out]
              }
            }
            n165 = Multiply(x=w339, y=w330) -> (x*y=w338:dbl)
            n166 = Add(x=w338, y=w337) -> (x+y=w333:dbl)
            n167 = case shown="True" w325 {
              tunnel: [enum16{"speed"}."speed" ("Enum") enum16{"speed"}."speed" ("Enum")] -> w331
              tunnel: [w346 w353] -> w332
              tunnel: w334 -> [w346 _]
              tunnel: w333 -> [_ w349]
              tunnel: w330 -> [_ w351]
              frame False {
              }
              frame True {
                n168 = Multiply(x=w351, y=-1.0) -> (x*y=w348:dbl)
                n169 = local write "Å]YÄ²1"(w349) -> ()
                n170 = Wait (ms)(milliseconds to wait=u32 25) -> ()  [unwired: 1 out]
                n171 = local write "Å]Vy1"(w348) -> ()
                n172 = Tick Count (ms)() -> (millisecond timer value=w353:u32)
              }
            }
            n173 = property on="魔王1" class="Bool (strict)"("Top"=w333) -> ()  [unwired: 2 in, 2 out]
            n174 = Wait (ms)(milliseconds to wait=u32 10) -> ()  [unwired: 1 out]
            n175 = property on="魔王1" class="Bool (strict)"() -> ("Top"=w315:i32)  [unwired: 2 in, 2 out]
          }
        }
        n176 = case shown="\"speed\"" w140 {
          tunnel: w141 -> [w287]
          tunnel: [w285] -> w139
          tunnel: [w284] -> w138
          tunnel: [w268] -> w137
          tunnel: w136 -> [w267]
          tunnel: w136 -> [w266]
          tunnel: w135 -> [w265]
          tunnel: w135 -> [w264]
          frame "speed" {
            n177 = Tick Count (ms)() -> (millisecond timer value=w296:u32)
            n178 = property on="魔王1" class="Bool (strict)"() -> ("Left"=w288:i32)  [unwired: 2 in, 2 out]
            n179 = property on="魔王1" class="Bool (strict)"() -> ("Left"=w282:i32)  [unwired: 2 in, 2 out]
            n180 = Less?(x=w282, y=0) -> (x < y?=w280:bool)
            n181 = Greater?(x=w267, y=500.0) -> (0:w262:bool)
            n182 = Greater?(x=w265, y=500.0) -> (0:w271:bool)
            n183 = Less?(x=w266, y=0.0) -> (x < y?=w274:bool)
            n184 = Less?(x=w264, y=0.0) -> (x < y?=w275:bool)
            n185 = Greater?(x=w288, y=500) -> (0:w279:bool)
            n186 = Subtract(x=w296, y=w287) -> (x-y=w295:u32)
            n187 = Or(x=w279, y=w280) -> (x .or. y?=w278:bool)
            n188 = To Double Precision Float(number=w295) -> (double precision float=w294:dbl)
            n189 = And(x=w262, y=w271) -> (x .and. y?=w276:bool)
            n190 = And(x=w274, y=w275) -> (x .and. y?=w277:bool)
            n191 = local read "Å]Vx1"() -> (w283:i32)
            n192 = Or(x=w276, y=w277) -> (x .or. y?=w263:bool)
            n193 = Divide(x=w294, y=1000.0) -> (x/y=w292:dbl)
            n194 = local read "Å]XÄ²1"() -> (w290:i32)
            n195 = case shown="True" w263 {
              frame False {
              }
              frame True {
                w297 = 200 ("x觸及位置")
                n196 = local write "Å]XÄ²1"(w297) -> ()
                n197 = Wait (ms)(milliseconds to wait=u32 100) -> ()  [unwired: 1 out]
                n198 = property on="魔王1" class="Bool (strict)"("Left"=w297) -> ()  [unwired: 2 in, 2 out]
              }
            }
            n199 = Multiply(x=w292, y=w283) -> (x*y=w291:dbl)
            n200 = Add(x=w291, y=w290) -> (x+y=w286:dbl)
            n201 = case shown="True" w278 {
              tunnel: [enum16{"speed"}."speed" ("Enum") enum16{"speed"}."speed" ("Enum")] -> w284
              tunnel: [w299 w306] -> w285
              tunnel: w287 -> [w299 _]
              tunnel: w286 -> [_ w302]
              tunnel: w283 -> [_ w304]
              frame False {
              }
              frame True {
                n202 = Multiply(x=w304, y=-1.0) -> (x*y=w301:dbl)
                n203 = local write "Å]XÄ²1"(w302) -> ()
                n204 = Wait (ms)(milliseconds to wait=u32 25) -> ()  [unwired: 1 out]
                n205 = local write "Å]Vx1"(w301) -> ()
                n206 = Tick Count (ms)() -> (millisecond timer value=w306:u32)
              }
            }
            n207 = property on="魔王1" class="Bool (strict)"("Left"=w286) -> ()  [unwired: 2 in, 2 out]
            n208 = Wait (ms)(milliseconds to wait=u32 10) -> ()  [unwired: 1 out]
            n209 = property on="魔王1" class="Bool (strict)"() -> ("Left"=w268:i32)  [unwired: 2 in, 2 out]
          }
        }
        n210 = Increment(x=w201) -> (x+1=w200:i32)
        n211 = property on="X障礙 2" class="Bool (strict)"() -> ("Top"=w151:i32)  [unwired: 2 in, 2 out]
        n212 = property on="X障礙 2" class="Bool (strict)"() -> ("Top"=w157:i32)  [unwired: 2 in, 2 out]
        n213 = property on="X障礙 2" class="Bool (strict)"() -> ("Left"=w164:i32)  [unwired: 2 in, 2 out]
        n214 = property on="X障礙 2" class="Bool (strict)"() -> ("Left"=w162:i32)  [unwired: 2 in, 2 out]
        n215 = call-poly <vilib>:"Acquire Input Data.vi"("device ID"=w256, "error in (no error)"=w255) -> ("device ID"=w223:refnum<k1>, "keys pressed"=w254:T1, "error out"=w222:errorcluster)  [unwired: 15 in]
        n216 = case shown="\"speed\"" w259 {
          tunnel: w260 -> [w540]
          tunnel: [w539] -> w258
          tunnel: [w538] -> w257
          tunnel: w242 -> [w520]
          tunnel: w242 -> [w519]
          tunnel: w241 -> [w518]
          tunnel: w241 -> [w517]
          tunnel: [w516] -> w245
          tunnel: w242 -> [_]
          tunnel: w241 -> [_]
          frame "speed" {
            n217 = Tick Count (ms)() -> (millisecond timer value=w549:u32)
            n218 = property on="Y障礙" class="Bool (strict)"() -> ("Top"=w541:i32)  [unwired: 2 in, 2 out]
            n219 = property on="Y障礙" class="Bool (strict)"() -> ("Top"=w535:i32)  [unwired: 2 in, 2 out]
            n220 = Less?(x=w535, y=0) -> (x < y?=w533:bool)
            n221 = Greater?(x=w541, y=400) -> (0:w532:bool)
            n222 = Subtract(x=w549, y=w540) -> (x-y=w548:u32)
            "x-y" <- w548
            n223 = Greater?(x=w520, y=400.0) -> (0:w526:bool)
            n224 = Greater?(x=w518, y=400.0) -> (0:w525:bool)
            n225 = Less?(x=w519, y=0.0) -> (x < y?=w522:bool)
            n226 = Less?(x=w517, y=0.0) -> (x < y?=w521:bool)
            n227 = Or(x=w532, y=w533) -> (x .or. y?=w531:bool)
            n228 = To Double Precision Float(number=w548) -> (double precision float=w547:dbl)
            n229 = And(x=w526, y=w525) -> (x .and. y?=w515:bool)
            n230 = And(x=w522, y=w521) -> (x .and. y?=w514:bool)
            n231 = local read "Vy"() -> (w537:i32)
            n232 = local read "y觸及位置"() -> (w543:i32)
            n233 = Divide(x=w547, y=1000.0) -> (x/y=w545:dbl)
            n234 = Compound Arithmetic op=OR(w515, w514) -> (w513:bool)
            n235 = case shown="True" w513 {
              frame False {
              }
              frame True {
                w550 = 200 ("y觸及位置")
                n236 = local write "y觸及位置"(w550) -> ()
                n237 = Wait (ms)(milliseconds to wait=u32 100) -> ()  [unwired: 1 out]
                n238 = property on="Y障礙" class="Bool (strict)"("Top"=w550) -> ()  [unwired: 2 in, 2 out]
              }
            }
            n239 = Multiply(x=w545, y=w537) -> (x*y=w544:dbl)
            n240 = Add(x=w544, y=w543) -> (x+y=w529:dbl)
            n241 = case shown="True" w531 {
              tunnel: [enum16{"speed"}."speed" ("Enum") enum16{"speed"}."speed" ("Enum")] -> w538
              tunnel: [w552 w559] -> w539
              tunnel: w540 -> [w552 _]
              tunnel: w529 -> [_ w555]
              tunnel: w537 -> [_ w557]
              frame False {
              }
              frame True {
                n242 = local write "y觸及位置"(w555) -> ()
                n243 = Multiply(x=w557, y=-1.0) -> (x*y=w554:dbl)
                n244 = Wait (ms)(milliseconds to wait=u32 25) -> ()  [unwired: 1 out]
                n245 = Tick Count (ms)() -> (millisecond timer value=w559:u32)
                n246 = local write "Vy"(w554) -> ()
              }
            }
            n247 = property on="Y障礙" class="Bool (strict)"("Top"=w529) -> ()  [unwired: 2 in, 2 out]
            n248 = Wait (ms)(milliseconds to wait=u32 10) -> ()  [unwired: 1 out]
            n249 = property on="Y障礙" class="Bool (strict)"() -> ("Top"=w516:i32, "Left"=→"x位置":i32)  [unwired: 2 in, 2 out]
            "Y位置" <- w516
          }
        }
        n250 = local write "遊玩時間"(w200) -> ()
        n251 = local read "Y"() -> (w165:dbl)
        n252 = local read "X"() -> (w166:dbl)
        n253 = Array To Cluster(array=w254) -> (cluster=w224:T2)
        n254 = Unbundle(w224) -> ("keys pressed[0]"=w253:T3)  [unwired: 8 out]
        n255 = case shown="\"A\"" w253 {
          frame Default {
          }
          frame "A" {
            n256 = local read "X"() -> (w511:dbl)
            n257 = Wait (ms)(milliseconds to wait=u32 10) -> ()  [unwired: 1 out]
            n258 = Add(x=-2.0, y=w511) -> (x+y=w509:dbl)
            n259 = local write "X"(w509) -> ()
            n260 = property on="小精靈" class="Bool (strict)"("Left"=w509) -> ()  [unwired: 2 in, 2 out]
          }
        }
        n261 = case shown="\"D\"" w253 {
          frame Default {
          }
          frame "D" {
            n262 = local read "X"() -> (w507:dbl)
            n263 = Wait (ms)(milliseconds to wait=u32 10) -> ()  [unwired: 1 out]
            n264 = Add(x=2.0, y=w507) -> (x+y=w505:dbl)
            n265 = local write "X"(w505) -> ()
            n266 = property on="小精靈" class="Bool (strict)"("Left"=w505) -> ()  [unwired: 2 in, 2 out]
          }
        }
        n267 = Greater?(x=w199, y=500) -> (0:w197:bool)
        n268 = Add(x=w164, y=17) -> (x+y=w159:i32)
        n269 = Subtract(x=w162, y=17) -> (x-y=w160:i32)
        n270 = Subtract(x=w157, y=15) -> (x-y=w156:i32)
        n271 = Greater?(x=w248, y=250) -> (0:w205:bool)
        n272 = Add(x=w151, y=20) -> (x+y=w152:i32)
        n273 = property on="X障礙" class="Bool (strict)"() -> ("Top"=w221:i32)  [unwired: 2 in, 2 out]
        n274 = property on="X障礙" class="Bool (strict)"() -> ("Top"=w215:i32)  [unwired: 2 in, 2 out]
        n275 = property on="X障礙" class="Bool (strict)"() -> ("Left"=w208:i32)  [unwired: 2 in, 2 out]
        n276 = property on="X障礙" class="Bool (strict)"() -> ("Left"=w210:i32)  [unwired: 2 in, 2 out]
        n277 = In Range and Coerce(upper limit=w159, x=w166, lower limit=w160) -> (In Range?=w155:bool)  [unwired: 1 out]
        n278 = In Range and Coerce(upper limit=w152, x=w165, lower limit=w156) -> (In Range?=w154:bool)  [unwired: 1 out]
        n279 = local read "Y"() -> (w207:dbl)
        n280 = local read "X"() -> (w206:dbl)
        n281 = And(x=w155, y=w154) -> (x .and. y?=w150:bool)
        n282 = Add(x=w208, y=17) -> (x+y=w213:i32)
        n283 = Subtract(x=w210, y=17) -> (x-y=w212:i32)
        n284 = Subtract(x=w215, y=15) -> (x-y=w216:i32)
        n285 = Add(x=w221, y=20) -> (x+y=w220:i32)
        n286 = property on="Y障礙 2" class="Bool (strict)"() -> ("Top"=w182:i32)  [unwired: 2 in, 2 out]
        n287 = property on="Y障礙 2" class="Bool (strict)"() -> ("Top"=w176:i32)  [unwired: 2 in, 2 out]
        n288 = property on="Y障礙 2" class="Bool (strict)"() -> ("Left"=w169:i32)  [unwired: 2 in, 2 out]
        n289 = property on="Y障礙 2" class="Bool (strict)"() -> ("Left"=w171:i32)  [unwired: 2 in, 2 out]
        n290 = In Range and Coerce(upper limit=w213, x=w206, lower limit=w212) -> (In Range?=w217:bool)  [unwired: 1 out]
        n291 = In Range and Coerce(upper limit=w220, x=w207, lower limit=w216) -> (In Range?=w218:bool)  [unwired: 1 out]
        n292 = local read "Y"() -> (w168:dbl)
        n293 = local read "X"() -> (w167:dbl)
        n294 = And(x=w217, y=w218) -> (x .and. y?=w203:bool)
        n295 = Add(x=w169, y=17) -> (x+y=w174:i32)
        n296 = Subtract(x=w171, y=17) -> (x-y=w173:i32)
        n297 = Subtract(x=w176, y=15) -> (x-y=w177:i32)
        n298 = Add(x=w182, y=20) -> (x+y=w181:i32)
        n299 = case shown="\"W\"" w253 {
          frame Default {
          }
          frame "W" {
            n300 = local read "Y"() -> (w503:dbl)
            n301 = Wait (ms)(milliseconds to wait=u32 10) -> ()  [unwired: 1 out]
            n302 = Add(x=-2.0, y=w503) -> (x+y=w501:dbl)
            n303 = local write "Y"(w501) -> ()
            n304 = property on="小精靈" class="Bool (strict)"("Top"=w501) -> ()  [unwired: 2 in, 2 out]
          }
        }
        n305 = case shown="\"S\"" w253 {
          frame Default {
          }
          frame "S" {
            n306 = local read "Y"() -> (w499:dbl)
            n307 = Wait (ms)(milliseconds to wait=u32 10) -> ()  [unwired: 1 out]
            n308 = Add(x=2.0, y=w499) -> (x+y=w497:dbl)
            n309 = local write "Y"(w497) -> ()
            n310 = property on="小精靈" class="Bool (strict)"("Top"=w497) -> ()  [unwired: 2 in, 2 out]
          }
        }
        n311 = property on="Y障礙" class="Bool (strict)"() -> ("Top"=w225:i32)  [unwired: 2 in, 2 out]
        n312 = property on="Y障礙" class="Bool (strict)"() -> ("Top"=w231:i32)  [unwired: 2 in, 2 out]
        n313 = property on="Y障礙" class="Bool (strict)"() -> ("Left"=w238:i32)  [unwired: 2 in, 2 out]
        n314 = property on="Y障礙" class="Bool (strict)"() -> ("Left"=w236:i32)  [unwired: 2 in, 2 out]
        n315 = property on="魔王1" class="Bool (strict)"() -> ("Top"=w121:i32)  [unwired: 2 in, 2 out]
        n316 = property on="魔王1" class="Bool (strict)"() -> ("Top"=w125:i32)  [unwired: 2 in, 2 out]
        n317 = property on="魔王1" class="Bool (strict)"() -> ("Left"=w132:i32)  [unwired: 2 in, 2 out]
        n318 = property on="魔王1" class="Bool (strict)"() -> ("Left"=w130:i32)  [unwired: 2 in, 2 out]
        n319 = local read "Y"() -> (w239:dbl)
        n320 = In Range and Coerce(upper limit=w174, x=w167, lower limit=w173) -> (In Range?=w178:bool)  [unwired: 1 out]
        n321 = In Range and Coerce(upper limit=w181, x=w168, lower limit=w177) -> (In Range?=w179:bool)  [unwired: 1 out]
        n322 = local read "X"() -> (w240:dbl)
        n323 = local read "Y"() -> (w133:dbl)
        n324 = local read "X"() -> (w134:dbl)
        n325 = And(x=w178, y=w179) -> (x .and. y?=w149:bool)
        n326 = Add(x=w238, y=17) -> (x+y=w233:i32)
        n327 = Subtract(x=w236, y=17) -> (x-y=w234:i32)
        n328 = Subtract(x=w231, y=15) -> (x-y=w230:i32)
        n329 = Add(x=w225, y=20) -> (x+y=w226:i32)
        n330 = Add(x=w132, y=17) -> (x+y=w127:i32)
        n331 = Subtract(x=w130, y=17) -> (x-y=w128:i32)
        n332 = Subtract(x=w125, y=15) -> (x-y=w124:i32)
        n333 = Add(x=w121, y=20) -> (x+y=w122:i32)
        n334 = In Range and Coerce(upper limit=w233, x=w240, lower limit=w234) -> (In Range?=w229:bool)  [unwired: 1 out]
        n335 = In Range and Coerce(upper limit=w226, x=w239, lower limit=w230) -> (In Range?=w228:bool)  [unwired: 1 out]
        n336 = In Range and Coerce(upper limit=w127, x=w134, lower limit=w128) -> (In Range?=w120:bool)  [unwired: 1 out]
        n337 = In Range and Coerce(upper limit=w122, x=w133, lower limit=w124) -> (In Range?=w119:bool)  [unwired: 1 out]
        n338 = And(x=w229, y=w228) -> (x .and. y?=w204:bool)
        n339 = And(x=w120, y=w119) -> (x .and. y?=w118:bool)
        n340 = Compound Arithmetic op=OR(w118, w197, w205, w203, w204, w150, w149) -> (w202:bool)
      }
      n341 = call-poly <vilib>:"Close Input Device.vi"("error in (no error)"=w112, "device ID"=w114) -> ()  [unwired: 8 in, 1 out]
    }
    frame #2 {
      w565 = 1 ("Position:Left")
      w577 = 0 ("x*y")
      n342 = Random Number (0-1)() -> (number: 0 to 1=w582:dbl)
      n343 = Random Number (0-1)() -> (number: 0 to 1=w586:dbl)
      n344 = property on="Y障礙" class="Bool (strict)"("Left"=375 ("Position:Left"), "Top"=1 ("Position:Top")) -> ()  [unwired: 2 in, 2 out]
      n345 = property on="Y障礙 2" class="Bool (strict)"("Left"=300 ("Position:Left"), "Top"=1 ("Position:Top")) -> ()  [unwired: 2 in, 2 out]
      n346 = property on="魔王1" class="Bool (strict)"("Left"=w565, "Top"=w565) -> ()  [unwired: 2 in, 2 out]
      n347 = local write "x觸及位置 2"(0 ("x觸及位置")) -> ()
      n348 = local write "Vy"(300 ("Vy")) -> ()
      n349 = local write "Vx"(300 ("Vx")) -> ()
      n350 = Multiply(x=200.0, y=w582) -> (x*y=w580:dbl)
      n351 = Add(x=300.0 ("y"), y=w580) -> (x+y=→"Å]Vy":dbl)
      n352 = local write "y觸及位置 2"(0 ("y觸及位置")) -> ()
      n353 = local write "y觸及位置"(0 ("y觸及位置")) -> ()
      n354 = local write "x觸及位置"(0 ("x觸及位置")) -> ()
      n355 = Multiply(x=200.0, y=w586) -> (x*y=w584:dbl)
      n356 = Add(x=300.0 ("y"), y=w584) -> (x+y=→"Å]Vx":dbl)
      n357 = local write "Å]XÄ²1"(0 ("Vy")) -> ()
      n358 = local write "Å]YÄ²1"(0 ("Vx")) -> ()
      n359 = property on="X障礙 2" class="Bool (strict)"("Left"=1 ("Position:Left"), "Top"=270 ("Position:Top")) -> ()  [unwired: 2 in, 2 out]
      n360 = local write "Å]Vy1"(470 ("Vx")) -> ()
      n361 = local write "Å]Vx1"(350 ("Vy")) -> ()
      n362 = property on="X障礙" class="Bool (strict)"("Left"=1 ("Position:Left"), "Top"=340 ("Position:Top")) -> ()  [unwired: 2 in, 2 out]
      n363 = local write "Vx 2"(300 ("Vx 2")) -> ()
      n364 = local write "Vy 2"(270 ("Vy 2")) -> ()
      "Å]XÄ²" <- w577
      "Å]YÄ²" <- w577
    }
    frame #3 {
      w599 = 0 ("Left")
      w602 = 0 ("Left")
      w614 = 0 ("Left")
      w613 = 0 ("Top")
      w624 = 0
      w625 = 0
      w634 = 0 ("Top")
      w635 = 0
      n365 = Tick Count (ms)() -> (millisecond timer value=w637:u32)
      n366 = Tick Count (ms)() -> (millisecond timer value=w601:u32)
      n367 = Tick Count (ms)() -> (millisecond timer value=w628:u32)
      n368 = Tick Count (ms)() -> (millisecond timer value=w617:u32)
      n369 = Tick Count (ms)() -> (millisecond timer value=w616:u32)
      n370 = Tick Count (ms)() -> (millisecond timer value=w604:u32)
      n371 = call <vilib>:"Intialize Keyboard.vi"() -> ("error out"=w638:errorcluster, "device ID"=w639:refnum<k1>)  [unwired: 10 in]
      n372 = Tick Count (ms)() -> (millisecond timer value=w627:u32)
      n373 = Tick Count (ms)() -> (millisecond timer value=w640:u32)
      n374 = while {
        shift-right: [w820] -> _
        shift-left: enum16{"speed"}."speed" ("Enum") -> [w822]
        shift-right: [w821] -> _
        shift-left: w640 -> [w823]
        tunnel: w639 -> [w819]
        tunnel: w638 -> [w818]
        shift-right: [w814] -> _
        shift-left: w637 -> [w815]
        shift-right: [w813] -> _
        shift-left: enum16{"speed"}."speed" ("Enum") -> [w812]
        shift-right: [w811] -> _
        shift-left: w635 -> [w810]
        shift-left: w635 -> [w809]
        shift-right: [w808] -> _
        shift-left: w634 -> [w807]
        shift-left: w634 -> [w806]
        tunnel: w633 -> [w729]
        tunnel: w632 -> [w728]
        tunnel: [w788] -> w631
        tunnel: [w787] -> w630
        shift-right: [w753] -> _
        shift-left: w625 -> [w755]
        shift-left: w625 -> [w754]
        shift-right: [w750] -> _
        shift-left: w624 -> [w751]
        shift-left: w624 -> [w752]
        shift-right: [w749] -> _
        shift-left: w628 -> [w758]
        shift-right: [w748] -> _
        shift-left: enum16{"speed"}."speed" ("Enum") -> [w759]
        shift-right: [w747] -> _
        shift-left: w627 -> [w757]
        shift-right: [w746] -> _
        shift-left: enum16{"speed"}."speed" ("Enum") -> [w756]
        tunnel: [w729] -> w623
        tunnel: [w728] -> w622
        tunnel: [w725] -> w619
        tunnel: [w726] -> w620
        tunnel: [w727] -> w621
        shift-right: [w720] -> _
        shift-left: w617 -> [w722]
        shift-right: [w721] -> _
        shift-left: enum16{"speed"}."speed" ("Enum") -> [w723]
        shift-right: [w719] -> _
        shift-left: w613 -> [w718]
        shift-left: w613 -> [w717]
        shift-right: [w714] -> _
        shift-left: w616 -> [w716]
        shift-right: [w713] -> _
        shift-left: enum16{"speed"}."speed" ("Enum") -> [w715]
        shift-right: [w712] -> _
        shift-left: w614 -> [w711]
        shift-left: w614 -> [w710]
        tunnel: [w709] -> w610
        tunnel: w612 -> [w709]
        tunnel: [w708] -> w609
        tunnel: w611 -> [w708]
        tunnel: [w675] -> w608
        tunnel: [w674] -> w607
        tunnel: w606 -> [w673]
        tunnel: [w673] -> w605
        shift-right: [w670] -> _
        shift-left: w604 -> [w672]
        shift-right: [w669] -> _
        shift-left: enum16{"speed"}."speed" ("Enum") -> [w671]
        shift-right: [w668] -> _
        shift-left: w602 -> [w667]
        shift-left: w602 -> [w666]
        shift-right: [w663] -> _
        shift-left: w601 -> [w665]
        shift-right: [w662] -> _
        shift-left: enum16{"speed"}."speed" ("Enum") -> [w664]
        shift-right: [w661] -> _
        shift-left: w599 -> [w660]
        shift-left: w599 -> [w659]
        tunnel: [w642] -> w598
        stop <- w770 stop-if-true
        # "假終點"
        # "以下雙方向障礙"
        n375 = local read "遊玩時間"() -> (w768:i32)
        n376 = case shown="\"speed\"" w812 {
          tunnel: w815 -> [w1132]
          tunnel: [w1130] -> w814
          tunnel: [w1129] -> w813
          tunnel: [w1113] -> w811
          tunnel: w810 -> [w1112]
          tunnel: w810 -> [w1111]
          tunnel: w809 -> [w1110]
          tunnel: w809 -> [w1109]
          frame "speed" {
            n377 = Tick Count (ms)() -> (millisecond timer value=w1141:u32)
            n378 = property on="X障礙" class="Bool (strict)"() -> ("Left"=w1133:i32)  [unwired: 2 in, 2 out]
            n379 = property on="X障礙" class="Bool (strict)"() -> ("Left"=w1127:i32)  [unwired: 2 in, 2 out]
            n380 = Less?(x=w1127, y=0) -> (x < y?=w1125:bool)
            n381 = Greater?(x=w1112, y=500.0) -> (0:w1107:bool)
            n382 = Greater?(x=w1110, y=500.0) -> (0:w1116:bool)
            n383 = Less?(x=w1111, y=0.0) -> (x < y?=w1119:bool)
            n384 = Less?(x=w1109, y=0.0) -> (x < y?=w1120:bool)
            n385 = Greater?(x=w1133, y=500) -> (0:w1124:bool)
            n386 = Subtract(x=w1141, y=w1132) -> (x-y=w1140:u32)
            n387 = Or(x=w1124, y=w1125) -> (x .or. y?=w1123:bool)
            n388 = To Double Precision Float(number=w1140) -> (double precision float=w1139:dbl)
            n389 = And(x=w1107, y=w1116) -> (x .and. y?=w1121:bool)
            n390 = And(x=w1119, y=w1120) -> (x .and. y?=w1122:bool)
            n391 = Or(x=w1121, y=w1122) -> (x .or. y?=w1108:bool)
            n392 = local read "Vx"() -> (w1128:i32)
            n393 = local read "x觸及位置"() -> (w1135:i32)
            n394 = Divide(x=w1139, y=1000.0) -> (x/y=w1137:dbl)
            n395 = case shown="True" w1108 {
              frame False {
              }
              frame True {
                w1142 = 200 ("x觸及位置")
                n396 = local write "x觸及位置"(w1142) -> ()
                n397 = Wait (ms)(milliseconds to wait=u32 100) -> ()  [unwired: 1 out]
                n398 = property on="X障礙" class="Bool (strict)"("Left"=w1142) -> ()  [unwired: 2 in, 2 out]
              }
            }
            n399 = Multiply(x=w1137, y=w1128) -> (x*y=w1136:dbl)
            n400 = Add(x=w1136, y=w1135) -> (x+y=w1131:dbl)
            n401 = case shown="True" w1123 {
              tunnel: [enum16{"speed"}."speed" ("Enum") enum16{"speed"}."speed" ("Enum")] -> w1129
              tunnel: [w1144 w1151] -> w1130
              tunnel: w1132 -> [w1144 _]
              tunnel: w1131 -> [_ w1147]
              tunnel: w1128 -> [_ w1149]
              frame False {
              }
              frame True {
                n402 = local write "x觸及位置"(w1147) -> ()
                n403 = Multiply(x=w1149, y=-1.0) -> (x*y=w1146:dbl)
                n404 = Wait (ms)(milliseconds to wait=u32 25) -> ()  [unwired: 1 out]
                n405 = Tick Count (ms)() -> (millisecond timer value=w1151:u32)
                n406 = local write "Vx"(w1146) -> ()
              }
            }
            n407 = property on="X障礙" class="Bool (strict)"("Left"=w1131) -> ()  [unwired: 2 in, 2 out]
            n408 = Wait (ms)(milliseconds to wait=u32 10) -> ()  [unwired: 1 out]
            n409 = property on="X障礙" class="Bool (strict)"() -> ("Left"=w1113:i32)  [unwired: 2 in, 2 out]
          }
        }
        n410 = case shown="\"speed\"" w723 {
          tunnel: w722 -> [w991]
          tunnel: [w989] -> w720
          tunnel: [w988] -> w721
          tunnel: [w972] -> w719
          tunnel: w718 -> [w971]
          tunnel: w718 -> [w970]
          tunnel: w717 -> [w969]
          tunnel: w717 -> [w968]
          frame "speed" {
            n411 = Tick Count (ms)() -> (millisecond timer value=w1000:u32)
            n412 = property on="Y障礙 2" class="Bool (strict)"() -> ("Top"=w992:i32)  [unwired: 2 in, 2 out]
            n413 = property on="Y障礙 2" class="Bool (strict)"() -> ("Top"=w986:i32)  [unwired: 2 in, 2 out]
            n414 = Less?(x=w986, y=0) -> (x < y?=w984:bool)
            n415 = Greater?(x=w971, y=400.0) -> (0:w966:bool)
            n416 = Greater?(x=w969, y=400.0) -> (0:w975:bool)
            n417 = Less?(x=w970, y=0.0) -> (x < y?=w978:bool)
            n418 = Less?(x=w968, y=0.0) -> (x < y?=w979:bool)
            n419 = Greater?(x=w992, y=400) -> (0:w983:bool)
            n420 = Subtract(x=w1000, y=w991) -> (x-y=w999:u32)
            n421 = Or(x=w983, y=w984) -> (x .or. y?=w982:bool)
            n422 = To Double Precision Float(number=w999) -> (double precision float=w998:dbl)
            n423 = And(x=w966, y=w975) -> (x .and. y?=w980:bool)
            n424 = And(x=w978, y=w979) -> (x .and. y?=w981:bool)
            n425 = Or(x=w980, y=w981) -> (x .or. y?=w967:bool)
            n426 = local read "Vy 2"() -> (w987:i32)
            n427 = local read "y觸及位置 2"() -> (w994:i32)
            n428 = Divide(x=w998, y=1000.0) -> (x/y=w996:dbl)
            n429 = case shown="True" w967 {
              frame False {
              }
              frame True {
                w1001 = 200 ("x觸及位置")
                n430 = local write "y觸及位置 2"(w1001) -> ()
                n431 = Wait (ms)(milliseconds to wait=u32 100) -> ()  [unwired: 1 out]
                n432 = property on="Y障礙 2" class="Bool (strict)"("Top"=w1001) -> ()  [unwired: 2 in, 2 out]
              }
            }
            n433 = Multiply(x=w996, y=w987) -> (x*y=w995:dbl)
            n434 = Add(x=w995, y=w994) -> (x+y=w990:dbl)
            n435 = case shown="True" w982 {
              tunnel: [enum16{"speed"}."speed" ("Enum") enum16{"speed"}."speed" ("Enum")] -> w988
              tunnel: [w1003 w1010] -> w989
              tunnel: w991 -> [w1003 _]
              tunnel: w990 -> [_ w1006]
              tunnel: w987 -> [_ w1008]
              frame False {
              }
              frame True {
                n436 = local write "y觸及位置 2"(w1006) -> ()
                n437 = Multiply(x=w1008, y=-1.0) -> (x*y=w1005:dbl)
                n438 = Wait (ms)(milliseconds to wait=u32 25) -> ()  [unwired: 1 out]
                n439 = local write "Vy 2"(w1005) -> ()
                n440 = Tick Count (ms)() -> (millisecond timer value=w1010:u32)
              }
            }
            n441 = property on="Y障礙 2" class="Bool (strict)"("Top"=w990) -> ()  [unwired: 2 in, 2 out]
            n442 = Wait (ms)(milliseconds to wait=u32 10) -> ()  [unwired: 1 out]
            n443 = property on="Y障礙 2" class="Bool (strict)"() -> ("Top"=w972:i32)  [unwired: 2 in, 2 out]
          }
        }
        n444 = case shown="\"speed\"" w759 {
          tunnel: w758 -> [w1085]
          tunnel: [w1083] -> w749
          tunnel: [w1082] -> w748
          tunnel: [w1066] -> w753
          tunnel: w755 -> [w1065]
          tunnel: w755 -> [w1064]
          tunnel: w754 -> [w1063]
          tunnel: w754 -> [w1062]
          frame "speed" {
            n445 = Tick Count (ms)() -> (millisecond timer value=w1094:u32)
            n446 = property on="魔王" class="Bool (strict)"() -> ("Left"=w1086:i32)  [unwired: 2 in, 2 out]
            n447 = property on="魔王" class="Bool (strict)"() -> ("Left"=w1080:i32)  [unwired: 2 in, 2 out]
            n448 = Less?(x=w1080, y=0) -> (x < y?=w1078:bool)
            n449 = Greater?(x=w1065, y=500.0) -> (0:w1060:bool)
            n450 = Greater?(x=w1063, y=500.0) -> (0:w1069:bool)
            n451 = Less?(x=w1064, y=0.0) -> (x < y?=w1072:bool)
            n452 = Less?(x=w1062, y=0.0) -> (x < y?=w1073:bool)
            n453 = Greater?(x=w1086, y=500) -> (0:w1077:bool)
            n454 = Subtract(x=w1094, y=w1085) -> (x-y=w1093:u32)
            n455 = Or(x=w1077, y=w1078) -> (x .or. y?=w1076:bool)
            n456 = To Double Precision Float(number=w1093) -> (double precision float=w1092:dbl)
            n457 = And(x=w1060, y=w1069) -> (x .and. y?=w1074:bool)
            n458 = And(x=w1072, y=w1073) -> (x .and. y?=w1075:bool)
            n459 = Or(x=w1074, y=w1075) -> (x .or. y?=w1061:bool)
            n460 = local read "Å]Vx"() -> (w1081:i32)
            n461 = Divide(x=w1092, y=1000.0) -> (x/y=w1090:dbl)
            n462 = local read "Å]XÄ²"() -> (w1088:i32)
            n463 = case shown="True" w1061 {
              frame False {
              }
              frame True {
                w1095 = 200 ("x觸及位置")
                n464 = local write "Å]XÄ²"(w1095) -> ()
                n465 = Wait (ms)(milliseconds to wait=u32 100) -> ()  [unwired: 1 out]
                n466 = property on="魔王" class="Bool (strict)"("Left"=w1095) -> ()  [unwired: 2 in, 2 out]
              }
            }
            n467 = Multiply(x=w1090, y=w1081) -> (x*y=w1089:dbl)
            n468 = Add(x=w1089, y=w1088) -> (x+y=w1084:dbl)
            n469 = case shown="True" w1076 {
              tunnel: [enum16{"speed"}."speed" ("Enum") enum16{"speed"}."speed" ("Enum")] -> w1082
              tunnel: [w1097 w1104] -> w1083
              tunnel: w1085 -> [w1097 _]
              tunnel: w1084 -> [_ w1100]
              tunnel: w1081 -> [_ w1102]
              frame False {
              }
              frame True {
                n470 = Multiply(x=w1102, y=-1.0) -> (x*y=w1099:dbl)
                n471 = local write "Å]XÄ²"(w1100) -> ()
                n472 = Wait (ms)(milliseconds to wait=u32 25) -> ()  [unwired: 1 out]
                n473 = local write "Å]Vx"(w1099) -> ()
                n474 = Tick Count (ms)() -> (millisecond timer value=w1104:u32)
              }
            }
            n475 = property on="魔王" class="Bool (strict)"("Left"=w1084) -> ()  [unwired: 2 in, 2 out]
            n476 = Wait (ms)(milliseconds to wait=u32 10) -> ()  [unwired: 1 out]
            n477 = property on="魔王" class="Bool (strict)"() -> ("Left"=w1066:i32)  [unwired: 2 in, 2 out]
          }
        }
        n478 = case shown="\"speed\"" w756 {
          tunnel: w757 -> [w1038]
          tunnel: [w1036] -> w747
          tunnel: [w1035] -> w746
          tunnel: [w1019] -> w750
          tunnel: w752 -> [w1018]
          tunnel: w752 -> [w1017]
          tunnel: w751 -> [w1016]
          tunnel: w751 -> [w1015]
          frame "speed" {
            n479 = Tick Count (ms)() -> (millisecond timer value=w1047:u32)
            n480 = property on="魔王" class="Bool (strict)"() -> ("Top"=w1039:i32)  [unwired: 2 in, 2 out]
            n481 = property on="魔王" class="Bool (strict)"() -> ("Top"=w1033:i32)  [unwired: 2 in, 2 out]
            n482 = Less?(x=w1033, y=0) -> (x < y?=w1031:bool)
            n483 = Greater?(x=w1018, y=400.0) -> (0:w1013:bool)
            n484 = Greater?(x=w1016, y=400.0) -> (0:w1022:bool)
            n485 = Less?(x=w1017, y=0.0) -> (x < y?=w1025:bool)
            n486 = Less?(x=w1015, y=0.0) -> (x < y?=w1026:bool)
            n487 = Greater?(x=w1039, y=400) -> (0:w1030:bool)
            n488 = Subtract(x=w1047, y=w1038) -> (x-y=w1046:u32)
            n489 = Or(x=w1030, y=w1031) -> (x .or. y?=w1029:bool)
            n490 = To Double Precision Float(number=w1046) -> (double precision float=w1045:dbl)
            n491 = And(x=w1013, y=w1022) -> (x .and. y?=w1027:bool)
            n492 = And(x=w1025, y=w1026) -> (x .and. y?=w1028:bool)
            n493 = Or(x=w1027, y=w1028) -> (x .or. y?=w1014:bool)
            n494 = local read "Å]Vy"() -> (w1034:i64)
            n495 = Divide(x=w1045, y=1000.0) -> (x/y=w1043:dbl)
            n496 = local read "Å]YÄ²"() -> (w1041:i32)
            n497 = case shown="True" w1014 {
              frame False {
              }
              frame True {
                w1048 = 200 ("x觸及位置")
                n498 = local write "Å]YÄ²"(w1048) -> ()
                n499 = Wait (ms)(milliseconds to wait=u32 100) -> ()  [unwired: 1 out]
                n500 = property on="魔王" class="Bool (strict)"("Top"=w1048) -> ()  [unwired: 2 in, 2 out]
              }
            }
            n501 = Multiply(x=w1043, y=w1034) -> (x*y=w1042:dbl)
            n502 = Add(x=w1042, y=w1041) -> (x+y=w1037:dbl)
            n503 = case shown="True" w1029 {
              tunnel: [enum16{"speed"}."speed" ("Enum") enum16{"speed"}."speed" ("Enum")] -> w1035
              tunnel: [w1050 w1057] -> w1036
              tunnel: w1038 -> [w1050 _]
              tunnel: w1037 -> [_ w1053]
              tunnel: w1034 -> [_ w1055]
              frame False {
              }
              frame True {
                n504 = Multiply(x=w1055, y=-1.0) -> (x*y=w1052:dbl)
                n505 = local write "Å]YÄ²"(w1053) -> ()
                n506 = Wait (ms)(milliseconds to wait=u32 25) -> ()  [unwired: 1 out]
                n507 = local write "Å]Vy"(w1052) -> ()
                n508 = Tick Count (ms)() -> (millisecond timer value=w1057:u32)
              }
            }
            n509 = property on="魔王" class="Bool (strict)"("Top"=w1037) -> ()  [unwired: 2 in, 2 out]
            n510 = Wait (ms)(milliseconds to wait=u32 10) -> ()  [unwired: 1 out]
            n511 = property on="魔王" class="Bool (strict)"() -> ("Top"=w1019:i32)  [unwired: 2 in, 2 out]
          }
        }
        n512 = case shown="\"speed\"" w671 {
          tunnel: w672 -> [w897]
          tunnel: [w895] -> w670
          tunnel: [w894] -> w669
          tunnel: [w878] -> w668
          tunnel: w667 -> [w877]
          tunnel: w667 -> [w876]
          tunnel: w666 -> [w875]
          tunnel: w666 -> [w874]
          frame "speed" {
            n513 = Tick Count (ms)() -> (millisecond timer value=w906:u32)
            n514 = property on="魔王1" class="Bool (strict)"() -> ("Left"=w898:i32)  [unwired: 2 in, 2 out]
            n515 = property on="魔王1" class="Bool (strict)"() -> ("Left"=w892:i32)  [unwired: 2 in, 2 out]
            n516 = Less?(x=w892, y=0) -> (x < y?=w890:bool)
            n517 = Greater?(x=w877, y=500.0) -> (0:w872:bool)
            n518 = Greater?(x=w875, y=500.0) -> (0:w881:bool)
            n519 = Less?(x=w876, y=0.0) -> (x < y?=w884:bool)
            n520 = Less?(x=w874, y=0.0) -> (x < y?=w885:bool)
            n521 = Greater?(x=w898, y=500) -> (0:w889:bool)
            n522 = Subtract(x=w906, y=w897) -> (x-y=w905:u32)
            n523 = Or(x=w889, y=w890) -> (x .or. y?=w888:bool)
            n524 = To Double Precision Float(number=w905) -> (double precision float=w904:dbl)
            n525 = And(x=w872, y=w881) -> (x .and. y?=w886:bool)
            n526 = And(x=w884, y=w885) -> (x .and. y?=w887:bool)
            n527 = local read "Å]Vx1"() -> (w893:i32)
            n528 = Or(x=w886, y=w887) -> (x .or. y?=w873:bool)
            n529 = Divide(x=w904, y=1000.0) -> (x/y=w902:dbl)
            n530 = local read "Å]XÄ²1"() -> (w900:i32)
            n531 = case shown="True" w873 {
              frame False {
              }
              frame True {
                w907 = 200 ("x觸及位置")
                n532 = local write "Å]XÄ²1"(w907) -> ()
                n533 = Wait (ms)(milliseconds to wait=u32 100) -> ()  [unwired: 1 out]
                n534 = property on="魔王1" class="Bool (strict)"("Left"=w907) -> ()  [unwired: 2 in, 2 out]
              }
            }
            n535 = Multiply(x=w902, y=w893) -> (x*y=w901:dbl)
            n536 = Add(x=w901, y=w900) -> (x+y=w896:dbl)
            n537 = case shown="True" w888 {
              tunnel: [enum16{"speed"}."speed" ("Enum") enum16{"speed"}."speed" ("Enum")] -> w894
              tunnel: [w909 w916] -> w895
              tunnel: w897 -> [w909 _]
              tunnel: w896 -> [_ w912]
              tunnel: w893 -> [_ w914]
              frame False {
              }
              frame True {
                n538 = Multiply(x=w914, y=-1.0) -> (x*y=w911:dbl)
                n539 = local write "Å]XÄ²1"(w912) -> ()
                n540 = Wait (ms)(milliseconds to wait=u32 25) -> ()  [unwired: 1 out]
                n541 = local write "Å]Vx1"(w911) -> ()
                n542 = Tick Count (ms)() -> (millisecond timer value=w916:u32)
              }
            }
            n543 = property on="魔王1" class="Bool (strict)"("Left"=w896) -> ()  [unwired: 2 in, 2 out]
            n544 = Wait (ms)(milliseconds to wait=u32 10) -> ()  [unwired: 1 out]
            n545 = property on="魔王1" class="Bool (strict)"() -> ("Left"=w878:i32)  [unwired: 2 in, 2 out]
          }
        }
        n546 = case shown="\"speed\"" w664 {
          tunnel: w665 -> [w850]
          tunnel: [w848] -> w663
          tunnel: [w847] -> w662
          tunnel: [w831] -> w661
          tunnel: w660 -> [w830]
          tunnel: w660 -> [w829]
          tunnel: w659 -> [w828]
          tunnel: w659 -> [w827]
          frame "speed" {
            n547 = Tick Count (ms)() -> (millisecond timer value=w859:u32)
            n548 = property on="魔王1" class="Bool (strict)"() -> ("Top"=w851:i32)  [unwired: 2 in, 2 out]
            n549 = property on="魔王1" class="Bool (strict)"() -> ("Top"=w845:i32)  [unwired: 2 in, 2 out]
            n550 = Less?(x=w845, y=0) -> (x < y?=w843:bool)
            n551 = Greater?(x=w830, y=400.0) -> (0:w825:bool)
            n552 = Greater?(x=w828, y=400.0) -> (0:w834:bool)
            n553 = Less?(x=w829, y=0.0) -> (x < y?=w837:bool)
            n554 = Less?(x=w827, y=0.0) -> (x < y?=w838:bool)
            n555 = Greater?(x=w851, y=400) -> (0:w842:bool)
            n556 = Subtract(x=w859, y=w850) -> (x-y=w858:u32)
            n557 = Or(x=w842, y=w843) -> (x .or. y?=w841:bool)
            n558 = To Double Precision Float(number=w858) -> (double precision float=w857:dbl)
            n559 = And(x=w825, y=w834) -> (x .and. y?=w839:bool)
            n560 = And(x=w837, y=w838) -> (x .and. y?=w840:bool)
            n561 = local read "Å]Vy1"() -> (w846:i32)
            n562 = Or(x=w839, y=w840) -> (x .or. y?=w826:bool)
            n563 = Divide(x=w857, y=1000.0) -> (x/y=w855:dbl)
            n564 = local read "Å]YÄ²1"() -> (w853:i32)
            n565 = case shown="True" w826 {
              frame False {
              }
              frame True {
                w860 = 200 ("x觸及位置")
                n566 = local write "Å]YÄ²1"(w860) -> ()
                n567 = Wait (ms)(milliseconds to wait=u32 100) -> ()  [unwired: 1 out]
                n568 = property on="魔王1" class="Bool (strict)"("Top"=w860) -> ()  [unwired: 2 in, 2 out]
              }
            }
            n569 = Multiply(x=w855, y=w846) -> (x*y=w854:dbl)
            n570 = Add(x=w854, y=w853) -> (x+y=w849:dbl)
            n571 = case shown="True" w841 {
              tunnel: [enum16{"speed"}."speed" ("Enum") enum16{"speed"}."speed" ("Enum")] -> w847
              tunnel: [w862 w869] -> w848
              tunnel: w850 -> [w862 _]
              tunnel: w849 -> [_ w865]
              tunnel: w846 -> [_ w867]
              frame False {
              }
              frame True {
                n572 = Multiply(x=w867, y=-1.0) -> (x*y=w864:dbl)
                n573 = local write "Å]YÄ²1"(w865) -> ()
                n574 = Wait (ms)(milliseconds to wait=u32 25) -> ()  [unwired: 1 out]
                n575 = local write "Å]Vy1"(w864) -> ()
                n576 = Tick Count (ms)() -> (millisecond timer value=w869:u32)
              }
            }
            n577 = property on="魔王1" class="Bool (strict)"("Top"=w849) -> ()  [unwired: 2 in, 2 out]
            n578 = Wait (ms)(milliseconds to wait=u32 10) -> ()  [unwired: 1 out]
            n579 = property on="魔王1" class="Bool (strict)"() -> ("Top"=w831:i32)  [unwired: 2 in, 2 out]
          }
        }
        n580 = case shown="\"speed\"" w715 {
          tunnel: w716 -> [w944]
          tunnel: [w942] -> w714
          tunnel: [w941] -> w713
          tunnel: [w925] -> w712
          tunnel: w711 -> [w924]
          tunnel: w711 -> [w923]
          tunnel: w710 -> [w922]
          tunnel: w710 -> [w921]
          frame "speed" {
            n581 = Tick Count (ms)() -> (millisecond timer value=w953:u32)
            n582 = property on="X障礙 2" class="Bool (strict)"() -> ("Left"=w945:i32)  [unwired: 2 in, 2 out]
            n583 = property on="X障礙 2" class="Bool (strict)"() -> ("Left"=w939:i32)  [unwired: 2 in, 2 out]
            n584 = Less?(x=w939, y=0) -> (x < y?=w937:bool)
            n585 = Greater?(x=w924, y=500.0) -> (0:w919:bool)
            n586 = Greater?(x=w922, y=500.0) -> (0:w928:bool)
            n587 = Less?(x=w923, y=0.0) -> (x < y?=w931:bool)
            n588 = Less?(x=w921, y=0.0) -> (x < y?=w932:bool)
            n589 = Greater?(x=w945, y=500) -> (0:w936:bool)
            n590 = Subtract(x=w953, y=w944) -> (x-y=w952:u32)
            n591 = Or(x=w936, y=w937) -> (x .or. y?=w935:bool)
            n592 = To Double Precision Float(number=w952) -> (double precision float=w951:dbl)
            n593 = And(x=w919, y=w928) -> (x .and. y?=w933:bool)
            n594 = And(x=w931, y=w932) -> (x .and. y?=w934:bool)
            n595 = Or(x=w933, y=w934) -> (x .or. y?=w920:bool)
            n596 = local read "Vx 2"() -> (w940:i32)
            n597 = local read "x觸及位置 2"() -> (w947:i32)
            n598 = Divide(x=w951, y=1000.0) -> (x/y=w949:dbl)
            n599 = case shown="True" w920 {
              frame False {
              }
              frame True {
                w954 = 200 ("x觸及位置")
                n600 = local write "x觸及位置 2"(w954) -> ()
                n601 = Wait (ms)(milliseconds to wait=u32 100) -> ()  [unwired: 1 out]
                n602 = property on="X障礙 2" class="Bool (strict)"("Left"=w954) -> ()  [unwired: 2 in, 2 out]
              }
            }
            n603 = Multiply(x=w949, y=w940) -> (x*y=w948:dbl)
            n604 = Add(x=w948, y=w947) -> (x+y=w943:dbl)
            n605 = case shown="True" w935 {
              tunnel: [enum16{"speed"}."speed" ("Enum") enum16{"speed"}."speed" ("Enum")] -> w941
              tunnel: [w956 w963] -> w942
              tunnel: w944 -> [w956 _]
              tunnel: w943 -> [_ w959]
              tunnel: w940 -> [_ w961]
              frame False {
              }
              frame True {
                n606 = local write "x觸及位置 2"(w959) -> ()
                n607 = Multiply(x=w961, y=-1.0) -> (x*y=w958:dbl)
                n608 = Wait (ms)(milliseconds to wait=u32 25) -> ()  [unwired: 1 out]
                n609 = local write "Vx 2"(w958) -> ()
                n610 = Tick Count (ms)() -> (millisecond timer value=w963:u32)
              }
            }
            n611 = property on="X障礙 2" class="Bool (strict)"("Left"=w943) -> ()  [unwired: 2 in, 2 out]
            n612 = Wait (ms)(milliseconds to wait=u32 10) -> ()  [unwired: 1 out]
            n613 = property on="X障礙 2" class="Bool (strict)"() -> ("Left"=w925:i32)  [unwired: 2 in, 2 out]
          }
        }
        n614 = case shown="\"speed\"" w822 {
          tunnel: w823 -> [w1195]
          tunnel: [w1193] -> w821
          tunnel: [w1192] -> w820
          tunnel: [w1176] -> w808
          tunnel: w807 -> [w1175]
          tunnel: w807 -> [w1174]
          tunnel: w806 -> [w1173]
          tunnel: w806 -> [w1172]
          frame "speed" {
            n615 = Tick Count (ms)() -> (millisecond timer value=w1204:u32)
            n616 = Greater?(x=w1175, y=400.0) -> (0:w1170:bool)
            n617 = Greater?(x=w1173, y=400.0) -> (0:w1179:bool)
            n618 = Less?(x=w1174, y=0.0) -> (x < y?=w1182:bool)
            n619 = Less?(x=w1172, y=0.0) -> (x < y?=w1183:bool)
            n620 = property on="Y障礙" class="Bool (strict)"() -> ("Top"=w1196:i32)  [unwired: 2 in, 2 out]
            n621 = property on="Y障礙" class="Bool (strict)"() -> ("Top"=w1190:i32)  [unwired: 2 in, 2 out]
            n622 = Less?(x=w1190, y=0) -> (x < y?=w1188:bool)
            n623 = Greater?(x=w1196, y=400) -> (0:w1187:bool)
            n624 = Subtract(x=w1204, y=w1195) -> (x-y=w1203:u32)
            n625 = Or(x=w1187, y=w1188) -> (x .or. y?=w1186:bool)
            n626 = And(x=w1170, y=w1179) -> (x .and. y?=w1184:bool)
            n627 = And(x=w1182, y=w1183) -> (x .and. y?=w1185:bool)
            n628 = To Double Precision Float(number=w1203) -> (double precision float=w1202:dbl)
            n629 = Or(x=w1184, y=w1185) -> (x .or. y?=w1171:bool)
            n630 = local read "Vy"() -> (w1191:i32)
            n631 = local read "y觸及位置"() -> (w1198:i32)
            n632 = Divide(x=w1202, y=1000.0) -> (x/y=w1200:dbl)
            n633 = case shown="True" w1171 {
              frame False {
              }
              frame True {
                w1205 = 200 ("y觸及位置")
                n634 = local write "y觸及位置"(w1205) -> ()
                n635 = Wait (ms)(milliseconds to wait=u32 100) -> ()  [unwired: 1 out]
                n636 = property on="Y障礙" class="Bool (strict)"("Top"=w1205) -> ()  [unwired: 2 in, 2 out]
              }
            }
            n637 = Multiply(x=w1200, y=w1191) -> (x*y=w1199:dbl)
            n638 = Add(x=w1199, y=w1198) -> (x+y=w1194:dbl)
            n639 = case shown="True" w1186 {
              tunnel: [enum16{"speed"}."speed" ("Enum") enum16{"speed"}."speed" ("Enum")] -> w1192
              tunnel: [w1207 w1214] -> w1193
              tunnel: w1195 -> [w1207 _]
              tunnel: w1194 -> [_ w1210]
              tunnel: w1191 -> [_ w1212]
              frame False {
              }
              frame True {
                n640 = local write "y觸及位置"(w1210) -> ()
                n641 = Multiply(x=w1212, y=-1.0) -> (x*y=w1209:dbl)
                n642 = Wait (ms)(milliseconds to wait=u32 25) -> ()  [unwired: 1 out]
                n643 = Tick Count (ms)() -> (millisecond timer value=w1214:u32)
                n644 = local write "Vy"(w1209) -> ()
              }
            }
            n645 = property on="Y障礙" class="Bool (strict)"("Top"=w1194) -> ()  [unwired: 2 in, 2 out]
            n646 = property on="Y障礙" class="Bool (strict)"() -> ("Top"=w1176:i32)  [unwired: 2 in, 2 out]
            n647 = Wait (ms)(milliseconds to wait=u32 10) -> ()  [unwired: 1 out]
          }
        }
        n648 = call-poly <vilib>:"Acquire Input Data.vi"("device ID"=w819, "error in (no error)"=w818) -> ("device ID"=w788:refnum<k1>, "keys pressed"=w817:T1, "error out"=w787:errorcluster)  [unwired: 15 in]
        n649 = Increment(x=w768) -> (x+1=w769:i32)
        n650 = local write "遊玩時間"(w769) -> ()
        n651 = Array To Cluster(array=w817) -> (cluster=w805:T2)
        n652 = Unbundle(w805) -> ("keys pressed[0]"=w816:T3)  [unwired: 8 out]
        n653 = case shown="\"A\"" w816 {
          frame Default {
          }
          frame "A" {
            n654 = local read "X"() -> (w1167:dbl)
            n655 = Wait (ms)(milliseconds to wait=u32 10) -> ()  [unwired: 1 out]
            n656 = Add(x=-2.0, y=w1167) -> (x+y=w1165:dbl)
            n657 = local write "X"(w1165) -> ()
            n658 = property on="小精靈" class="Bool (strict)"("Left"=w1165) -> ()  [unwired: 2 in, 2 out]
          }
        }
        n659 = case shown="\"D\"" w816 {
          frame Default {
          }
          frame "D" {
            n660 = local read "X"() -> (w1163:dbl)
            n661 = Wait (ms)(milliseconds to wait=u32 10) -> ()  [unwired: 1 out]
            n662 = Add(x=2.0, y=w1163) -> (x+y=w1161:dbl)
            n663 = local write "X"(w1161) -> ()
            n664 = property on="小精靈" class="Bool (strict)"("Left"=w1161) -> ()  [unwired: 2 in, 2 out]
          }
        }
        n665 = property on="Y障礙" class="Bool (strict)"() -> ("Top"=w789:i32)  [unwired: 2 in, 2 out]
        n666 = property on="Y障礙" class="Bool (strict)"() -> ("Top"=w795:i32)  [unwired: 2 in, 2 out]
        n667 = property on="Y障礙" class="Bool (strict)"() -> ("Left"=w802:i32)  [unwired: 2 in, 2 out]
        n668 = property on="Y障礙" class="Bool (strict)"() -> ("Left"=w800:i32)  [unwired: 2 in, 2 out]
        n669 = case shown="\"W\"" w816 {
          frame Default {
          }
          frame "W" {
            n670 = local read "Y"() -> (w1159:dbl)
            n671 = Wait (ms)(milliseconds to wait=u32 10) -> ()  [unwired: 1 out]
            n672 = Add(x=-2.0, y=w1159) -> (x+y=w1157:dbl)
            n673 = local write "Y"(w1157) -> ()
            n674 = property on="小精靈" class="Bool (strict)"("Top"=w1157) -> ()  [unwired: 2 in, 2 out]
          }
        }
        n675 = case shown="\"S\"" w816 {
          frame Default {
          }
          frame "S" {
            n676 = local read "Y"() -> (w1155:dbl)
            n677 = Wait (ms)(milliseconds to wait=u32 10) -> ()  [unwired: 1 out]
            n678 = Add(x=2.0, y=w1155) -> (x+y=w1153:dbl)
            n679 = local write "Y"(w1153) -> ()
            n680 = property on="小精靈" class="Bool (strict)"("Top"=w1153) -> ()  [unwired: 2 in, 2 out]
          }
        }
        n681 = local read "Y"() -> (w803:dbl)
        n682 = local read "X"() -> (w804:dbl)
        n683 = Add(x=w802, y=17) -> (x+y=w797:i32)
        n684 = Subtract(x=w800, y=17) -> (x-y=w798:i32)
        n685 = Subtract(x=w795, y=15) -> (x-y=w794:i32)
        n686 = Add(x=w789, y=20) -> (x+y=w790:i32)
        n687 = In Range and Coerce(upper limit=w797, x=w804, lower limit=w798) -> (In Range?=w793:bool)  [unwired: 1 out]
        n688 = In Range and Coerce(upper limit=w790, x=w803, lower limit=w794) -> (In Range?=w792:bool)  [unwired: 1 out]
        n689 = And(x=w793, y=w792) -> (x .and. y?=w727:bool)
        n690 = property on="X障礙" class="Bool (strict)"() -> ("Top"=w786:i32)  [unwired: 2 in, 2 out]
        n691 = property on="X障礙" class="Bool (strict)"() -> ("Top"=w780:i32)  [unwired: 2 in, 2 out]
        n692 = property on="X障礙" class="Bool (strict)"() -> ("Left"=w773:i32)  [unwired: 2 in, 2 out]
        n693 = property on="X障礙" class="Bool (strict)"() -> ("Left"=w775:i32)  [unwired: 2 in, 2 out]
        n694 = local read "Y"() -> (w772:dbl)
        n695 = property on="魔王" class="Bool (strict)"() -> ("Top"=w730:i32)  [unwired: 2 in, 2 out]
        n696 = property on="魔王" class="Bool (strict)"() -> ("Top"=w736:i32)  [unwired: 2 in, 2 out]
        n697 = property on="魔王" class="Bool (strict)"() -> ("Left"=w743:i32)  [unwired: 2 in, 2 out]
        n698 = property on="魔王" class="Bool (strict)"() -> ("Left"=w741:i32)  [unwired: 2 in, 2 out]
        n699 = local read "X"() -> (w771:dbl)
        n700 = local read "X"() -> (w767:dbl)
        n701 = local read "Y"() -> (w766:dbl)
        n702 = property on="X障礙 2" class="Bool (strict)"() -> ("Top"=w707:i32)  [unwired: 2 in, 2 out]
        n703 = property on="X障礙 2" class="Bool (strict)"() -> ("Top"=w701:i32)  [unwired: 2 in, 2 out]
        n704 = property on="X障礙 2" class="Bool (strict)"() -> ("Left"=w694:i32)  [unwired: 2 in, 2 out]
        n705 = property on="X障礙 2" class="Bool (strict)"() -> ("Left"=w696:i32)  [unwired: 2 in, 2 out]
        n706 = property on="Y障礙 2" class="Bool (strict)"() -> ("Top"=w691:i32)  [unwired: 2 in, 2 out]
        n707 = property on="Y障礙 2" class="Bool (strict)"() -> ("Top"=w685:i32)  [unwired: 2 in, 2 out]
        n708 = property on="Y障礙 2" class="Bool (strict)"() -> ("Left"=w678:i32)  [unwired: 2 in, 2 out]
        n709 = property on="Y障礙 2" class="Bool (strict)"() -> ("Left"=w680:i32)  [unwired: 2 in, 2 out]
        n710 = local read "Y"() -> (w744:dbl)
        n711 = local read "X"() -> (w745:dbl)
        n712 = property on="魔王1" class="Bool (strict)"() -> ("Top"=w658:i32)  [unwired: 2 in, 2 out]
        n713 = property on="魔王1" class="Bool (strict)"() -> ("Top"=w652:i32)  [unwired: 2 in, 2 out]
        n714 = property on="魔王1" class="Bool (strict)"() -> ("Left"=w645:i32)  [unwired: 2 in, 2 out]
        n715 = property on="魔王1" class="Bool (strict)"() -> ("Left"=w647:i32)  [unwired: 2 in, 2 out]
        n716 = local read "Y"() -> (w693:dbl)
        n717 = local read "Y"() -> (w677:dbl)
        n718 = Add(x=w773, y=17) -> (x+y=w778:i32)
        n719 = Subtract(x=w775, y=17) -> (x-y=w777:i32)
        n720 = Subtract(x=w780, y=15) -> (x-y=w781:i32)
        n721 = local read "X"() -> (w692:dbl)
        n722 = local read "X"() -> (w676:dbl)
        n723 = Add(x=w786, y=20) -> (x+y=w785:i32)
        n724 = local read "Y"() -> (w644:dbl)
        n725 = In Range and Coerce(upper limit=516.0, x=w767, lower limit=463.0) -> (In Range?=w765:bool)  [unwired: 1 out]
        n726 = In Range and Coerce(upper limit=399.0, x=w766, lower limit=358.0) -> (In Range?=w764:bool)  [unwired: 1 out]
        n727 = local read "X"() -> (w643:dbl)
        n728 = Add(x=w743, y=17) -> (x+y=w738:i32)
        n729 = Subtract(x=w741, y=17) -> (x-y=w739:i32)
        n730 = Subtract(x=w736, y=15) -> (x-y=w735:i32)
        n731 = Add(x=w730, y=20) -> (x+y=w731:i32)
        n732 = Add(x=w694, y=17) -> (x+y=w699:i32)
        n733 = Subtract(x=w696, y=17) -> (x-y=w698:i32)
        n734 = Subtract(x=w701, y=15) -> (x-y=w702:i32)
        n735 = Add(x=w678, y=17) -> (x+y=w683:i32)
        n736 = Subtract(x=w680, y=17) -> (x-y=w682:i32)
        n737 = Subtract(x=w685, y=15) -> (x-y=w686:i32)
        n738 = In Range and Coerce(upper limit=w778, x=w771, lower limit=w777) -> (In Range?=w782:bool)  [unwired: 1 out]
        n739 = In Range and Coerce(upper limit=w785, x=w772, lower limit=w781) -> (In Range?=w783:bool)  [unwired: 1 out]
        n740 = Add(x=w707, y=20) -> (x+y=w706:i32)
        n741 = Add(x=w691, y=20) -> (x+y=w690:i32)
        n742 = And(x=w765, y=w764) -> (x .and. y?=w724:bool)
        n743 = Add(x=w645, y=17) -> (x+y=w650:i32)
        n744 = Subtract(x=w647, y=17) -> (x-y=w649:i32)
        n745 = Subtract(x=w652, y=15) -> (x-y=w653:i32)
        n746 = Add(x=w658, y=20) -> (x+y=w657:i32)
        n747 = In Range and Coerce(upper limit=w738, x=w745, lower limit=w739) -> (In Range?=w734:bool)  [unwired: 1 out]
        n748 = In Range and Coerce(upper limit=w731, x=w744, lower limit=w735) -> (In Range?=w733:bool)  [unwired: 1 out]
        n749 = And(x=w782, y=w783) -> (x .and. y?=w726:bool)
        n750 = In Range and Coerce(upper limit=w699, x=w692, lower limit=w698) -> (In Range?=w703:bool)  [unwired: 1 out]
        n751 = In Range and Coerce(upper limit=w706, x=w693, lower limit=w702) -> (In Range?=w704:bool)  [unwired: 1 out]
        n752 = In Range and Coerce(upper limit=w683, x=w676, lower limit=w682) -> (In Range?=w687:bool)  [unwired: 1 out]
        n753 = In Range and Coerce(upper limit=w690, x=w677, lower limit=w686) -> (In Range?=w688:bool)  [unwired: 1 out]
        n754 = In Range and Coerce(upper limit=w650, x=w643, lower limit=w649) -> (In Range?=w654:bool)  [unwired: 1 out]
        n755 = In Range and Coerce(upper limit=w657, x=w644, lower limit=w653) -> (In Range?=w655:bool)  [unwired: 1 out]
        n756 = And(x=w734, y=w733) -> (x .and. y?=w725:bool)
        n757 = And(x=w703, y=w704) -> (x .and. y?=w675:bool)
        n758 = And(x=w687, y=w688) -> (x .and. y?=w674:bool)
        n759 = And(x=w654, y=w655) -> (x .and. y?=w642:bool)
        n760 = Compound Arithmetic op=OR(w642, w673, w674, w675, w708, w709, w729, w728, w727, w726, w725, w724) -> (w770:bool)
      }
      n761 = call-poly <vilib>:"Close Input Device.vi"("error in (no error)"=w630, "device ID"=w631) -> ()  [unwired: 8 in, 1 out]
    }
    frame #4 {
      w1218 = 0 ("Å]YÄ²2")
      w1223 = 1 ("Position:Left")
      w1238 = 0 ("Position:Left")
      w1239 = 1 ("Position:Left")
      n762 = property on="Y障礙 2" class="Bool (strict)"("Left"=80 ("Position:Left"), "Top"=1 ("Position:Top")) -> ()  [unwired: 2 in, 2 out]
      n763 = property on="Y障礙" class="Bool (strict)"("Left"=375 ("Position:Left"), "Top"=1 ("Position:Top")) -> ()  [unwired: 2 in, 2 out]
      n764 = local write "x觸及位置 2"(0 ("x觸及位置")) -> ()
      n765 = property on="魔王1" class="Bool (strict)"("Left"=w1223, "Top"=w1223) -> ()  [unwired: 2 in, 2 out]
      n766 = property on="魔王" class="Bool (strict)"("Left"=w1239, "Top"=w1239) -> ()  [unwired: 2 in, 2 out]
      n767 = local write "y觸及位置 2"(0 ("y觸及位置")) -> ()
      n768 = local write "Vy"(400 ("Vy")) -> ()
      n769 = local write "Vx"(400 ("Vx")) -> ()
      n770 = local write "Å]Vy1"(470 ("Vx")) -> ()
      n771 = local write "y觸及位置"(0 ("y觸及位置")) -> ()
      n772 = local write "Å]Vx1"(350 ("Vy")) -> ()
      n773 = local write "x觸及位置"(0 ("x觸及位置")) -> ()
      n774 = local write "Å]XÄ²"(0 ("Vy")) -> ()
      n775 = local write "Å]Vx"(500 ("Vy")) -> ()
      n776 = local write "Å]Vy"(500 ("Vx")) -> ()
      n777 = local write "Å]YÄ²"(0 ("Vx")) -> ()
      n778 = local write "Å]XÄ²1"(0 ("Vy")) -> ()
      n779 = local write "Å]YÄ²1"(0 ("Vx")) -> ()
      n780 = property on="X障礙 2" class="Bool (strict)"("Left"=1 ("Position:Left"), "Top"=60 ("Position:Top")) -> ()  [unwired: 2 in, 2 out]
      n781 = local write "Vx 2"(350 ("Vx 2")) -> ()
      n782 = property on="X障礙" class="Bool (strict)"("Left"=1 ("Position:Left"), "Top"=340 ("Position:Top")) -> ()  [unwired: 2 in, 2 out]
      n783 = local write "Vy 2"(350 ("Vy 2")) -> ()
      n784 = property on="終點" class="Bool (strict)"("Left"=w1238, "Top"=w1238) -> ()  [unwired: 2 in, 2 out]
      "Å]XÄ²2" <- w1218
      "Å]Vx2" <- 300 ("Å]Vx2")
      "Å]YÄ²2" <- w1218
      "Å]Vy2" <- 200 ("Å]Vy2")
    }
    frame #5 {
      w1261 = 0 ("Left")
      w1264 = 0 ("Left")
      w1269 = 0 ("Left")
      w1272 = 0 ("Top")
      w1279 = 0 ("Top")
      w1284 = 0 ("Left")
      w1280 = 0 ("Left")
      w1291 = 0 ("Top")
      n785 = Tick Count (ms)() -> (millisecond timer value=w1265:u32)
      n786 = Tick Count (ms)() -> (millisecond timer value=w1260:u32)
      n787 = Tick Count (ms)() -> (millisecond timer value=w1287:u32)
      n788 = Tick Count (ms)() -> (millisecond timer value=w1282:u32)
      n789 = Tick Count (ms)() -> (millisecond timer value=w1271:u32)
      n790 = Tick Count (ms)() -> (millisecond timer value=w1263:u32)
      n791 = Tick Count (ms)() -> (millisecond timer value=w1285:u32)
      n792 = Tick Count (ms)() -> (millisecond timer value=w1274:u32)
      n793 = Tick Count (ms)() -> (millisecond timer value=w1258:u32)
      n794 = call <vilib>:"Intialize Keyboard.vi"() -> ("error out"=w1294:errorcluster, "device ID"=w1295:refnum<k1>)  [unwired: 10 in]
      n795 = Tick Count (ms)() -> (millisecond timer value=w1290:u32)
      n796 = while {
        shift-right: [w1516] -> _
        shift-left: enum16{"speed"}."speed" ("Enum") -> [w1518]
        shift-right: [w1517] -> _
        shift-left: w1290 -> [w1519]
        tunnel: w1295 -> [w1515]
        tunnel: w1294 -> [w1514]
        shift-right: [w1510] -> _
        shift-left: w1287 -> [w1511]
        shift-right: [w1509] -> _
        shift-left: enum16{"speed"}."speed" ("Enum") -> [w1508]
        shift-right: [w1507] -> _
        shift-left: w1291 -> [w1506]
        shift-left: w1291 -> [w1505]
        tunnel: [w1487] -> w1293
        tunnel: [w1486] -> w1292
        tunnel: [w1423] -> w1281
        shift-right: [w1452] -> _
        shift-left: w1284 -> [w1454]
        shift-left: w1284 -> [w1453]
        shift-right: [w1451] -> _
        shift-left: w1285 -> [w1457]
        shift-right: [w1450] -> _
        shift-left: enum16{"speed"}."speed" ("Enum") -> [w1458]
        shift-right: [w1449] -> _
        shift-left: w1282 -> [w1456]
        shift-right: [w1448] -> _
        shift-left: enum16{"speed"}."speed" ("Enum") -> [w1455]
        tunnel: w1300 -> [w1431]
        tunnel: w1299 -> [w1430]
        tunnel: w1298 -> [w1429]
        tunnel: w1297 -> [w1428]
        tunnel: w1296 -> [w1427]
        shift-right: [w1420] -> _
        shift-left: w1280 -> [w1422]
        shift-left: w1280 -> [w1421]
        shift-right: [w1417] -> _
        shift-left: w1279 -> [w1419]
        shift-left: w1279 -> [w1418]
        tunnel: w1278 -> [w1416]
        tunnel: w1277 -> [w1415]
        tunnel: w1276 -> [w1414]
        tunnel: w1275 -> [w1413]
        shift-right: [w1410] -> _
        shift-left: w1274 -> [w1412]
        shift-right: [w1409] -> _
        shift-left: enum16{"speed"}."speed" ("Enum") -> [w1411]
        shift-right: [w1408] -> _
        shift-left: w1272 -> [w1407]
        shift-left: w1272 -> [w1406]
        shift-right: [w1403] -> _
        shift-left: w1271 -> [w1405]
        shift-right: [w1402] -> _
        shift-left: enum16{"speed"}."speed" ("Enum") -> [w1404]
        shift-right: [w1401] -> _
        shift-left: w1269 -> [w1400]
        shift-left: w1269 -> [w1399]
        tunnel: w1268 -> [w1364]
        tunnel: w1267 -> [w1363]
        shift-right: [w1360] -> _
        shift-left: w1265 -> [w1361]
        shift-right: [w1359] -> _
        shift-left: enum16{"speed"}."speed" ("Enum") -> [w1362]
        shift-right: [w1358] -> _
        shift-left: w1264 -> [w1357]
        shift-left: w1264 -> [w1356]
        shift-right: [w1353] -> _
        shift-left: w1263 -> [w1355]
        shift-right: [w1352] -> _
        shift-left: enum16{"speed"}."speed" ("Enum") -> [w1354]
        shift-right: [w1351] -> _
        shift-left: w1261 -> [w1350]
        shift-left: w1261 -> [w1349]
        shift-right: [w1329] -> _
        shift-left: w1260 -> [w1331]
        shift-right: [w1328] -> _
        shift-left: enum16{"speed"}."speed" ("Enum") -> [w1330]
        shift-right: [w1327] -> _
        shift-left: _ -> [w1326]
        shift-left: _ -> [w1325]
        shift-right: [w1322] -> _
        shift-left: w1258 -> [w1324]
        shift-right: [w1321] -> _
        shift-left: enum16{"speed"}."speed" ("Enum") -> [w1323]
        shift-right: [w1320] -> _
        shift-left: _ -> [w1319]
        shift-left: _ -> [w1318]
        stop <- w1469 stop-if-true
        # "終點"
        # "以下雙方向障礙"
        n797 = local read "遊玩時間"() -> (w1467:i32)
        n798 = case shown="\"speed\"" w1508 {
          tunnel: w1511 -> [w1922]
          tunnel: [w1920] -> w1510
          tunnel: [w1919] -> w1509
          tunnel: [w1903] -> w1420
          tunnel: w1422 -> [w1902]
          tunnel: w1422 -> [w1901]
          tunnel: w1421 -> [w1900]
          tunnel: w1421 -> [w1899]
          frame "speed" {
            n799 = Tick Count (ms)() -> (millisecond timer value=w1931:u32)
            n800 = property on="X障礙" class="Bool (strict)"() -> ("Left"=w1923:i32)  [unwired: 2 in, 2 out]
            n801 = property on="X障礙" class="Bool (strict)"() -> ("Left"=w1917:i32)  [unwired: 2 in, 2 out]
            n802 = Less?(x=w1917, y=0) -> (x < y?=w1915:bool)
            n803 = Greater?(x=w1902, y=500.0) -> (0:w1897:bool)
            n804 = Greater?(x=w1900, y=500.0) -> (0:w1906:bool)
            n805 = Less?(x=w1901, y=0.0) -> (x < y?=w1909:bool)
            n806 = Less?(x=w1899, y=0.0) -> (x < y?=w1910:bool)
            n807 = Greater?(x=w1923, y=500) -> (0:w1914:bool)
            n808 = Subtract(x=w1931, y=w1922) -> (x-y=w1930:u32)
            n809 = Or(x=w1914, y=w1915) -> (x .or. y?=w1913:bool)
            n810 = To Double Precision Float(number=w1930) -> (double precision float=w1929:dbl)
            n811 = And(x=w1897, y=w1906) -> (x .and. y?=w1911:bool)
            n812 = And(x=w1909, y=w1910) -> (x .and. y?=w1912:bool)
            n813 = Or(x=w1911, y=w1912) -> (x .or. y?=w1898:bool)
            n814 = local read "Vx"() -> (w1918:i32)
            n815 = local read "x觸及位置"() -> (w1925:i32)
            n816 = Divide(x=w1929, y=1000.0) -> (x/y=w1927:dbl)
            n817 = case shown="True" w1898 {
              frame False {
              }
              frame True {
                w1932 = 200 ("x觸及位置")
                n818 = local write "x觸及位置"(w1932) -> ()
                n819 = Wait (ms)(milliseconds to wait=u32 100) -> ()  [unwired: 1 out]
                n820 = property on="X障礙" class="Bool (strict)"("Left"=w1932) -> ()  [unwired: 2 in, 2 out]
              }
            }
            n821 = Multiply(x=w1927, y=w1918) -> (x*y=w1926:dbl)
            n822 = Add(x=w1926, y=w1925) -> (x+y=w1921:dbl)
            n823 = case shown="True" w1913 {
              tunnel: [enum16{"speed"}."speed" ("Enum") enum16{"speed"}."speed" ("Enum")] -> w1919
              tunnel: [w1934 w1941] -> w1920
              tunnel: w1922 -> [w1934 _]
              tunnel: w1921 -> [_ w1937]
              tunnel: w1918 -> [_ w1939]
              frame False {
              }
              frame True {
                n824 = local write "x觸及位置"(w1937) -> ()
                n825 = Multiply(x=w1939, y=-1.0) -> (x*y=w1936:dbl)
                n826 = Wait (ms)(milliseconds to wait=u32 25) -> ()  [unwired: 1 out]
                n827 = Tick Count (ms)() -> (millisecond timer value=w1941:u32)
                n828 = local write "Vx"(w1936) -> ()
              }
            }
            n829 = property on="X障礙" class="Bool (strict)"("Left"=w1921) -> ()  [unwired: 2 in, 2 out]
            n830 = Wait (ms)(milliseconds to wait=u32 10) -> ()  [unwired: 1 out]
            n831 = property on="X障礙" class="Bool (strict)"() -> ("Left"=w1903:i32)  [unwired: 2 in, 2 out]
          }
        }
        n832 = case shown="\"speed\"" w1458 {
          tunnel: w1457 -> [w1875]
          tunnel: [w1873] -> w1451
          tunnel: [w1872] -> w1450
          tunnel: [w1856] -> w1452
          tunnel: w1454 -> [w1855]
          tunnel: w1454 -> [w1854]
          tunnel: w1453 -> [w1853]
          tunnel: w1453 -> [w1852]
          frame "speed" {
            n833 = Tick Count (ms)() -> (millisecond timer value=w1884:u32)
            n834 = property on="魔王" class="Bool (strict)"() -> ("Left"=w1876:i32)  [unwired: 2 in, 2 out]
            n835 = property on="魔王" class="Bool (strict)"() -> ("Left"=w1870:i32)  [unwired: 2 in, 2 out]
            n836 = Less?(x=w1870, y=0) -> (x < y?=w1868:bool)
            n837 = Greater?(x=w1855, y=500.0) -> (0:w1850:bool)
            n838 = Greater?(x=w1853, y=500.0) -> (0:w1859:bool)
            n839 = Less?(x=w1854, y=0.0) -> (x < y?=w1862:bool)
            n840 = Less?(x=w1852, y=0.0) -> (x < y?=w1863:bool)
            n841 = Greater?(x=w1876, y=500) -> (0:w1867:bool)
            n842 = Subtract(x=w1884, y=w1875) -> (x-y=w1883:u32)
            n843 = Or(x=w1867, y=w1868) -> (x .or. y?=w1866:bool)
            n844 = To Double Precision Float(number=w1883) -> (double precision float=w1882:dbl)
            n845 = And(x=w1850, y=w1859) -> (x .and. y?=w1864:bool)
            n846 = And(x=w1862, y=w1863) -> (x .and. y?=w1865:bool)
            n847 = Or(x=w1864, y=w1865) -> (x .or. y?=w1851:bool)
            n848 = local read "Å]Vx"() -> (w1871:i32)
            n849 = Divide(x=w1882, y=1000.0) -> (x/y=w1880:dbl)
            n850 = local read "Å]XÄ²"() -> (w1878:i32)
            n851 = case shown="True" w1851 {
              frame False {
              }
              frame True {
                w1885 = 200 ("x觸及位置")
                n852 = local write "Å]XÄ²"(w1885) -> ()
                n853 = Wait (ms)(milliseconds to wait=u32 100) -> ()  [unwired: 1 out]
                n854 = property on="魔王" class="Bool (strict)"("Left"=w1885) -> ()  [unwired: 2 in, 2 out]
              }
            }
            n855 = Multiply(x=w1880, y=w1871) -> (x*y=w1879:dbl)
            n856 = Add(x=w1879, y=w1878) -> (x+y=w1874:dbl)
            n857 = case shown="True" w1866 {
              tunnel: [enum16{"speed"}."speed" ("Enum") enum16{"speed"}."speed" ("Enum")] -> w1872
              tunnel: [w1887 w1894] -> w1873
              tunnel: w1875 -> [w1887 _]
              tunnel: w1874 -> [_ w1890]
              tunnel: w1871 -> [_ w1892]
              frame False {
              }
              frame True {
                n858 = Multiply(x=w1892, y=-1.0) -> (x*y=w1889:dbl)
                n859 = local write "Å]XÄ²"(w1890) -> ()
                n860 = Wait (ms)(milliseconds to wait=u32 25) -> ()  [unwired: 1 out]
                n861 = local write "Å]Vx"(w1889) -> ()
                n862 = Tick Count (ms)() -> (millisecond timer value=w1894:u32)
              }
            }
            n863 = property on="魔王" class="Bool (strict)"("Left"=w1874) -> ()  [unwired: 2 in, 2 out]
            n864 = Wait (ms)(milliseconds to wait=u32 10) -> ()  [unwired: 1 out]
            n865 = property on="魔王" class="Bool (strict)"() -> ("Left"=w1856:i32)  [unwired: 2 in, 2 out]
          }
        }
        n866 = case shown="\"speed\"" w1354 {
          tunnel: w1355 -> [w1640]
          tunnel: [w1638] -> w1353
          tunnel: [w1637] -> w1352
          tunnel: [w1621] -> w1351
          tunnel: w1350 -> [w1620]
          tunnel: w1350 -> [w1619]
          tunnel: w1349 -> [w1618]
          tunnel: w1349 -> [w1617]
          frame "speed" {
            n867 = Tick Count (ms)() -> (millisecond timer value=w1649:u32)
            n868 = property on="魔王1" class="Bool (strict)"() -> ("Top"=w1641:i32)  [unwired: 2 in, 2 out]
            n869 = property on="魔王1" class="Bool (strict)"() -> ("Top"=w1635:i32)  [unwired: 2 in, 2 out]
            n870 = Less?(x=w1635, y=0) -> (x < y?=w1633:bool)
            n871 = Greater?(x=w1620, y=400.0) -> (0:w1615:bool)
            n872 = Greater?(x=w1618, y=400.0) -> (0:w1624:bool)
            n873 = Less?(x=w1619, y=0.0) -> (x < y?=w1627:bool)
            n874 = Less?(x=w1617, y=0.0) -> (x < y?=w1628:bool)
            n875 = Greater?(x=w1641, y=400) -> (0:w1632:bool)
            n876 = Subtract(x=w1649, y=w1640) -> (x-y=w1648:u32)
            n877 = Or(x=w1632, y=w1633) -> (x .or. y?=w1631:bool)
            n878 = To Double Precision Float(number=w1648) -> (double precision float=w1647:dbl)
            n879 = And(x=w1615, y=w1624) -> (x .and. y?=w1629:bool)
            n880 = And(x=w1627, y=w1628) -> (x .and. y?=w1630:bool)
            n881 = local read "Å]Vy1"() -> (w1636:i32)
            n882 = Or(x=w1629, y=w1630) -> (x .or. y?=w1616:bool)
            n883 = Divide(x=w1647, y=1000.0) -> (x/y=w1645:dbl)
            n884 = local read "Å]YÄ²1"() -> (w1643:i32)
            n885 = case shown="True" w1616 {
              frame False {
              }
              frame True {
                w1650 = 200 ("x觸及位置")
                n886 = local write "Å]YÄ²1"(w1650) -> ()
                n887 = Wait (ms)(milliseconds to wait=u32 100) -> ()  [unwired: 1 out]
                n888 = property on="魔王1" class="Bool (strict)"("Top"=w1650) -> ()  [unwired: 2 in, 2 out]
              }
            }
            n889 = Multiply(x=w1645, y=w1636) -> (x*y=w1644:dbl)
            n890 = Add(x=w1644, y=w1643) -> (x+y=w1639:dbl)
            n891 = case shown="True" w1631 {
              tunnel: [enum16{"speed"}."speed" ("Enum") enum16{"speed"}."speed" ("Enum")] -> w1637
              tunnel: [w1652 w1659] -> w1638
              tunnel: w1640 -> [w1652 _]
              tunnel: w1639 -> [_ w1655]
              tunnel: w1636 -> [_ w1657]
              frame False {
              }
              frame True {
                n892 = Multiply(x=w1657, y=-1.0) -> (x*y=w1654:dbl)
                n893 = local write "Å]YÄ²1"(w1655) -> ()
                n894 = Wait (ms)(milliseconds to wait=u32 25) -> ()  [unwired: 1 out]
                n895 = local write "Å]Vy1"(w1654) -> ()
                n896 = Tick Count (ms)() -> (millisecond timer value=w1659:u32)
              }
            }
            n897 = property on="魔王1" class="Bool (strict)"("Top"=w1639) -> ()  [unwired: 2 in, 2 out]
            n898 = Wait (ms)(milliseconds to wait=u32 10) -> ()  [unwired: 1 out]
            n899 = property on="魔王1" class="Bool (strict)"() -> ("Top"=w1621:i32)  [unwired: 2 in, 2 out]
          }
        }
        n900 = case shown="\"speed\"" w1330 {
          tunnel: w1331 -> [w1593]
          tunnel: [w1591] -> w1329
          tunnel: [w1590] -> w1328
          tunnel: [w1574] -> w1327
          tunnel: w1326 -> [w1573]
          tunnel: w1326 -> [w1572]
          tunnel: w1325 -> [w1571]
          tunnel: w1325 -> [w1570]
          frame "speed" {
            n901 = Tick Count (ms)() -> (millisecond timer value=w1602:u32)
            n902 = property on="魔王2" class="Bool (strict)"() -> ("Top"=w1594:i32)  [unwired: 2 in, 2 out]
            n903 = property on="魔王2" class="Bool (strict)"() -> ("Top"=w1588:i32)  [unwired: 2 in, 2 out]
            n904 = Less?(x=w1588, y=0) -> (x < y?=w1586:bool)
            n905 = Greater?(x=w1573, y=400.0) -> (0:w1568:bool)
            n906 = Greater?(x=w1571, y=400.0) -> (0:w1577:bool)
            n907 = Less?(x=w1572, y=0.0) -> (x < y?=w1580:bool)
            n908 = Less?(x=w1570, y=0.0) -> (x < y?=w1581:bool)
            n909 = Greater?(x=w1594, y=400) -> (0:w1585:bool)
            n910 = Subtract(x=w1602, y=w1593) -> (x-y=w1601:u32)
            n911 = Or(x=w1585, y=w1586) -> (x .or. y?=w1584:bool)
            n912 = To Double Precision Float(number=w1601) -> (double precision float=w1600:dbl)
            n913 = And(x=w1568, y=w1577) -> (x .and. y?=w1582:bool)
            n914 = And(x=w1580, y=w1581) -> (x .and. y?=w1583:bool)
            n915 = local read "Å]Vy2"() -> (w1589:i32)
            n916 = Or(x=w1582, y=w1583) -> (x .or. y?=w1569:bool)
            n917 = Divide(x=w1600, y=1000.0) -> (x/y=w1598:dbl)
            n918 = local read "Å]YÄ²2"() -> (w1596:i32)
            n919 = case shown="True" w1569 {
              frame False {
              }
              frame True {
                w1603 = 200 ("x觸及位置")
                n920 = local write "Å]YÄ²2"(w1603) -> ()
                n921 = Wait (ms)(milliseconds to wait=u32 100) -> ()  [unwired: 1 out]
                n922 = property on="魔王2" class="Bool (strict)"("Top"=w1603) -> ()  [unwired: 2 in, 2 out]
              }
            }
            n923 = Multiply(x=w1598, y=w1589) -> (x*y=w1597:dbl)
            n924 = Add(x=w1597, y=w1596) -> (x+y=w1592:dbl)
            n925 = case shown="True" w1584 {
              tunnel: [enum16{"speed"}."speed" ("Enum") enum16{"speed"}."speed" ("Enum")] -> w1590
              tunnel: [w1605 w1612] -> w1591
              tunnel: w1593 -> [w1605 _]
              tunnel: w1592 -> [_ w1608]
              tunnel: w1589 -> [_ w1610]
              frame False {
              }
              frame True {
                n926 = Multiply(x=w1610, y=-1.0) -> (x*y=w1607:dbl)
                n927 = local write "Å]YÄ²2"(w1608) -> ()
                n928 = Wait (ms)(milliseconds to wait=u32 25) -> ()  [unwired: 1 out]
                n929 = local write "Å]Vy2"(w1607) -> ()
                n930 = Tick Count (ms)() -> (millisecond timer value=w1612:u32)
              }
            }
            n931 = property on="魔王2" class="Bool (strict)"("Top"=w1592) -> ()  [unwired: 2 in, 2 out]
            n932 = Wait (ms)(milliseconds to wait=u32 10) -> ()  [unwired: 1 out]
            n933 = property on="魔王2" class="Bool (strict)"() -> ("Top"=w1574:i32)  [unwired: 2 in, 2 out]
          }
        }
        n934 = case shown="\"speed\"" w1455 {
          tunnel: w1456 -> [w1828]
          tunnel: [w1826] -> w1449
          tunnel: [w1825] -> w1448
          tunnel: [w1809] -> w1417
          tunnel: w1419 -> [w1808]
          tunnel: w1419 -> [w1807]
          tunnel: w1418 -> [w1806]
          tunnel: w1418 -> [w1805]
          frame "speed" {
            n935 = Tick Count (ms)() -> (millisecond timer value=w1837:u32)
            n936 = property on="魔王" class="Bool (strict)"() -> ("Top"=w1829:i32)  [unwired: 2 in, 2 out]
            n937 = property on="魔王" class="Bool (strict)"() -> ("Top"=w1823:i32)  [unwired: 2 in, 2 out]
            n938 = Less?(x=w1823, y=0) -> (x < y?=w1821:bool)
            n939 = Greater?(x=w1808, y=400.0) -> (0:w1803:bool)
            n940 = Greater?(x=w1806, y=400.0) -> (0:w1812:bool)
            n941 = Less?(x=w1807, y=0.0) -> (x < y?=w1815:bool)
            n942 = Less?(x=w1805, y=0.0) -> (x < y?=w1816:bool)
            n943 = Greater?(x=w1829, y=400) -> (0:w1820:bool)
            n944 = Subtract(x=w1837, y=w1828) -> (x-y=w1836:u32)
            n945 = Or(x=w1820, y=w1821) -> (x .or. y?=w1819:bool)
            n946 = To Double Precision Float(number=w1836) -> (double precision float=w1835:dbl)
            n947 = And(x=w1803, y=w1812) -> (x .and. y?=w1817:bool)
            n948 = And(x=w1815, y=w1816) -> (x .and. y?=w1818:bool)
            n949 = Or(x=w1817, y=w1818) -> (x .or. y?=w1804:bool)
            n950 = local read "Å]Vy"() -> (w1824:i64)
            n951 = Divide(x=w1835, y=1000.0) -> (x/y=w1833:dbl)
            n952 = local read "Å]YÄ²"() -> (w1831:i32)
            n953 = case shown="True" w1804 {
              frame False {
              }
              frame True {
                w1838 = 200 ("x觸及位置")
                n954 = local write "Å]YÄ²"(w1838) -> ()
                n955 = Wait (ms)(milliseconds to wait=u32 100) -> ()  [unwired: 1 out]
                n956 = property on="魔王" class="Bool (strict)"("Top"=w1838) -> ()  [unwired: 2 in, 2 out]
              }
            }
            n957 = Multiply(x=w1833, y=w1824) -> (x*y=w1832:dbl)
            n958 = Add(x=w1832, y=w1831) -> (x+y=w1827:dbl)
            n959 = case shown="True" w1819 {
              tunnel: [enum16{"speed"}."speed" ("Enum") enum16{"speed"}."speed" ("Enum")] -> w1825
              tunnel: [w1840 w1847] -> w1826
              tunnel: w1828 -> [w1840 _]
              tunnel: w1827 -> [_ w1843]
              tunnel: w1824 -> [_ w1845]
              frame False {
              }
              frame True {
                n960 = Multiply(x=w1845, y=-1.0) -> (x*y=w1842:dbl)
                n961 = local write "Å]YÄ²"(w1843) -> ()
                n962 = Wait (ms)(milliseconds to wait=u32 25) -> ()  [unwired: 1 out]
                n963 = local write "Å]Vy"(w1842) -> ()
                n964 = Tick Count (ms)() -> (millisecond timer value=w1847:u32)
              }
            }
            n965 = property on="魔王" class="Bool (strict)"("Top"=w1827) -> ()  [unwired: 2 in, 2 out]
            n966 = Wait (ms)(milliseconds to wait=u32 10) -> ()  [unwired: 1 out]
            n967 = property on="魔王" class="Bool (strict)"() -> ("Top"=w1809:i32)  [unwired: 2 in, 2 out]
          }
        }
        n968 = case shown="\"speed\"" w1411 {
          tunnel: w1412 -> [w1781]
          tunnel: [w1779] -> w1410
          tunnel: [w1778] -> w1409
          tunnel: [w1762] -> w1408
          tunnel: w1407 -> [w1761]
          tunnel: w1407 -> [w1760]
          tunnel: w1406 -> [w1759]
          tunnel: w1406 -> [w1758]
          frame "speed" {
            n969 = Tick Count (ms)() -> (millisecond timer value=w1790:u32)
            n970 = property on="Y障礙 2" class="Bool (strict)"() -> ("Top"=w1782:i32)  [unwired: 2 in, 2 out]
            n971 = property on="Y障礙 2" class="Bool (strict)"() -> ("Top"=w1776:i32)  [unwired: 2 in, 2 out]
            n972 = Less?(x=w1776, y=0) -> (x < y?=w1774:bool)
            n973 = Greater?(x=w1761, y=400.0) -> (0:w1756:bool)
            n974 = Greater?(x=w1759, y=400.0) -> (0:w1765:bool)
            n975 = Less?(x=w1760, y=0.0) -> (x < y?=w1768:bool)
            n976 = Less?(x=w1758, y=0.0) -> (x < y?=w1769:bool)
            n977 = Greater?(x=w1782, y=400) -> (0:w1773:bool)
            n978 = Subtract(x=w1790, y=w1781) -> (x-y=w1789:u32)
            n979 = Or(x=w1773, y=w1774) -> (x .or. y?=w1772:bool)
            n980 = To Double Precision Float(number=w1789) -> (double precision float=w1788:dbl)
            n981 = And(x=w1756, y=w1765) -> (x .and. y?=w1770:bool)
            n982 = And(x=w1768, y=w1769) -> (x .and. y?=w1771:bool)
            n983 = Or(x=w1770, y=w1771) -> (x .or. y?=w1757:bool)
            n984 = local read "Vy 2"() -> (w1777:i32)
            n985 = local read "y觸及位置 2"() -> (w1784:i32)
            n986 = Divide(x=w1788, y=1000.0) -> (x/y=w1786:dbl)
            n987 = case shown="True" w1757 {
              frame False {
              }
              frame True {
                w1791 = 200 ("x觸及位置")
                n988 = local write "y觸及位置 2"(w1791) -> ()
                n989 = Wait (ms)(milliseconds to wait=u32 100) -> ()  [unwired: 1 out]
                n990 = property on="Y障礙 2" class="Bool (strict)"("Top"=w1791) -> ()  [unwired: 2 in, 2 out]
              }
            }
            n991 = Multiply(x=w1786, y=w1777) -> (x*y=w1785:dbl)
            n992 = Add(x=w1785, y=w1784) -> (x+y=w1780:dbl)
            n993 = case shown="True" w1772 {
              tunnel: [enum16{"speed"}."speed" ("Enum") enum16{"speed"}."speed" ("Enum")] -> w1778
              tunnel: [w1793 w1800] -> w1779
              tunnel: w1781 -> [w1793 _]
              tunnel: w1780 -> [_ w1796]
              tunnel: w1777 -> [_ w1798]
              frame False {
              }
              frame True {
                n994 = local write "y觸及位置 2"(w1796) -> ()
                n995 = Multiply(x=w1798, y=-1.0) -> (x*y=w1795:dbl)
                n996 = Wait (ms)(milliseconds to wait=u32 25) -> ()  [unwired: 1 out]
                n997 = local write "Vy 2"(w1795) -> ()
                n998 = Tick Count (ms)() -> (millisecond timer value=w1800:u32)
              }
            }
            n999 = property on="Y障礙 2" class="Bool (strict)"("Top"=w1780) -> ()  [unwired: 2 in, 2 out]
            n1000 = Wait (ms)(milliseconds to wait=u32 10) -> ()  [unwired: 1 out]
            n1001 = property on="Y障礙 2" class="Bool (strict)"() -> ("Top"=w1762:i32)  [unwired: 2 in, 2 out]
          }
        }
        n1002 = case shown="\"speed\"" w1404 {
          tunnel: w1405 -> [w1734]
          tunnel: [w1732] -> w1403
          tunnel: [w1731] -> w1402
          tunnel: [w1715] -> w1401
          tunnel: w1400 -> [w1714]
          tunnel: w1400 -> [w1713]
          tunnel: w1399 -> [w1712]
          tunnel: w1399 -> [w1711]
          frame "speed" {
            n1003 = Tick Count (ms)() -> (millisecond timer value=w1743:u32)
            n1004 = property on="X障礙 2" class="Bool (strict)"() -> ("Left"=w1735:i32)  [unwired: 2 in, 2 out]
            n1005 = property on="X障礙 2" class="Bool (strict)"() -> ("Left"=w1729:i32)  [unwired: 2 in, 2 out]
            n1006 = Less?(x=w1729, y=0) -> (x < y?=w1727:bool)
            n1007 = Greater?(x=w1714, y=500.0) -> (0:w1709:bool)
            n1008 = Greater?(x=w1712, y=500.0) -> (0:w1718:bool)
            n1009 = Less?(x=w1713, y=0.0) -> (x < y?=w1721:bool)
            n1010 = Less?(x=w1711, y=0.0) -> (x < y?=w1722:bool)
            n1011 = Greater?(x=w1735, y=500) -> (0:w1726:bool)
            n1012 = Subtract(x=w1743, y=w1734) -> (x-y=w1742:u32)
            n1013 = Or(x=w1726, y=w1727) -> (x .or. y?=w1725:bool)
            n1014 = To Double Precision Float(number=w1742) -> (double precision float=w1741:dbl)
            n1015 = And(x=w1709, y=w1718) -> (x .and. y?=w1723:bool)
            n1016 = And(x=w1721, y=w1722) -> (x .and. y?=w1724:bool)
            n1017 = Or(x=w1723, y=w1724) -> (x .or. y?=w1710:bool)
            n1018 = local read "Vx 2"() -> (w1730:i32)
            n1019 = local read "x觸及位置 2"() -> (w1737:i32)
            n1020 = Divide(x=w1741, y=1000.0) -> (x/y=w1739:dbl)
            n1021 = case shown="True" w1710 {
              frame False {
              }
              frame True {
                w1744 = 200 ("x觸及位置")
                n1022 = local write "x觸及位置 2"(w1744) -> ()
                n1023 = Wait (ms)(milliseconds to wait=u32 100) -> ()  [unwired: 1 out]
                n1024 = property on="X障礙 2" class="Bool (strict)"("Left"=w1744) -> ()  [unwired: 2 in, 2 out]
              }
            }
            n1025 = Multiply(x=w1739, y=w1730) -> (x*y=w1738:dbl)
            n1026 = Add(x=w1738, y=w1737) -> (x+y=w1733:dbl)
            n1027 = case shown="True" w1725 {
              tunnel: [enum16{"speed"}."speed" ("Enum") enum16{"speed"}."speed" ("Enum")] -> w1731
              tunnel: [w1746 w1753] -> w1732
              tunnel: w1734 -> [w1746 _]
              tunnel: w1733 -> [_ w1749]
              tunnel: w1730 -> [_ w1751]
              frame False {
              }
              frame True {
                n1028 = local write "x觸及位置 2"(w1749) -> ()
                n1029 = Multiply(x=w1751, y=-1.0) -> (x*y=w1748:dbl)
                n1030 = Wait (ms)(milliseconds to wait=u32 25) -> ()  [unwired: 1 out]
                n1031 = local write "Vx 2"(w1748) -> ()
                n1032 = Tick Count (ms)() -> (millisecond timer value=w1753:u32)
              }
            }
            n1033 = property on="X障礙 2" class="Bool (strict)"("Left"=w1733) -> ()  [unwired: 2 in, 2 out]
            n1034 = Wait (ms)(milliseconds to wait=u32 10) -> ()  [unwired: 1 out]
            n1035 = property on="X障礙 2" class="Bool (strict)"() -> ("Left"=w1715:i32)  [unwired: 2 in, 2 out]
          }
        }
        n1036 = case shown="\"speed\"" w1323 {
          tunnel: w1324 -> [w1546]
          tunnel: [w1544] -> w1322
          tunnel: [w1543] -> w1321
          tunnel: [w1527] -> w1320
          tunnel: w1319 -> [w1526]
          tunnel: w1319 -> [w1525]
          tunnel: w1318 -> [w1524]
          tunnel: w1318 -> [w1523]
          frame "speed" {
            n1037 = Tick Count (ms)() -> (millisecond timer value=w1555:u32)
            n1038 = property on="魔王2" class="Bool (strict)"() -> ("Left"=w1547:i32)  [unwired: 2 in, 2 out]
            n1039 = property on="魔王2" class="Bool (strict)"() -> ("Left"=w1541:i32)  [unwired: 2 in, 2 out]
            n1040 = Less?(x=w1541, y=0) -> (x < y?=w1539:bool)
            n1041 = Greater?(x=w1526, y=500.0) -> (0:w1521:bool)
            n1042 = Greater?(x=w1524, y=500.0) -> (0:w1530:bool)
            n1043 = Less?(x=w1525, y=0.0) -> (x < y?=w1533:bool)
            n1044 = Less?(x=w1523, y=0.0) -> (x < y?=w1534:bool)
            n1045 = Greater?(x=w1547, y=500) -> (0:w1538:bool)
            n1046 = Subtract(x=w1555, y=w1546) -> (x-y=w1554:u32)
            n1047 = Or(x=w1538, y=w1539) -> (x .or. y?=w1537:bool)
            n1048 = To Double Precision Float(number=w1554) -> (double precision float=w1553:dbl)
            n1049 = And(x=w1521, y=w1530) -> (x .and. y?=w1535:bool)
            n1050 = And(x=w1533, y=w1534) -> (x .and. y?=w1536:bool)
            n1051 = local read "Å]Vx2"() -> (w1542:i32)
            n1052 = Or(x=w1535, y=w1536) -> (x .or. y?=w1522:bool)
            n1053 = Divide(x=w1553, y=1000.0) -> (x/y=w1551:dbl)
            n1054 = local read "Å]XÄ²2"() -> (w1549:i32)
            n1055 = case shown="True" w1522 {
              frame False {
              }
              frame True {
                w1556 = 200 ("x觸及位置")
                n1056 = local write "Å]XÄ²2"(w1556) -> ()
                n1057 = Wait (ms)(milliseconds to wait=u32 100) -> ()  [unwired: 1 out]
                n1058 = property on="魔王2" class="Bool (strict)"("Left"=w1556) -> ()  [unwired: 2 in, 2 out]
              }
            }
            n1059 = Multiply(x=w1551, y=w1542) -> (x*y=w1550:dbl)
            n1060 = Add(x=w1550, y=w1549) -> (x+y=w1545:dbl)
            n1061 = case shown="True" w1537 {
              tunnel: [enum16{"speed"}."speed" ("Enum") enum16{"speed"}."speed" ("Enum")] -> w1543
              tunnel: [w1558 w1565] -> w1544
              tunnel: w1546 -> [w1558 _]
              tunnel: w1545 -> [_ w1561]
              tunnel: w1542 -> [_ w1563]
              frame False {
              }
              frame True {
                n1062 = Multiply(x=w1563, y=-1.0) -> (x*y=w1560:dbl)
                n1063 = local write "Å]XÄ²2"(w1561) -> ()
                n1064 = Wait (ms)(milliseconds to wait=u32 25) -> ()  [unwired: 1 out]
                n1065 = local write "Å]Vx2"(w1560) -> ()
                n1066 = Tick Count (ms)() -> (millisecond timer value=w1565:u32)
              }
            }
            n1067 = property on="魔王2" class="Bool (strict)"("Left"=w1545) -> ()  [unwired: 2 in, 2 out]
            n1068 = Wait (ms)(milliseconds to wait=u32 10) -> ()  [unwired: 1 out]
            n1069 = property on="魔王2" class="Bool (strict)"() -> ("Left"=w1527:i32)  [unwired: 2 in, 2 out]
          }
        }
        n1070 = case shown="\"speed\"" w1362 {
          tunnel: w1361 -> [w1687]
          tunnel: [w1685] -> w1360
          tunnel: [w1684] -> w1359
          tunnel: [w1668] -> w1358
          tunnel: w1357 -> [w1667]
          tunnel: w1357 -> [w1666]
          tunnel: w1356 -> [w1665]
          tunnel: w1356 -> [w1664]
          frame "speed" {
            n1071 = Tick Count (ms)() -> (millisecond timer value=w1696:u32)
            n1072 = property on="魔王1" class="Bool (strict)"() -> ("Left"=w1688:i32)  [unwired: 2 in, 2 out]
            n1073 = property on="魔王1" class="Bool (strict)"() -> ("Left"=w1682:i32)  [unwired: 2 in, 2 out]
            n1074 = Less?(x=w1682, y=0) -> (x < y?=w1680:bool)
            n1075 = Greater?(x=w1667, y=500.0) -> (0:w1662:bool)
            n1076 = Greater?(x=w1665, y=500.0) -> (0:w1671:bool)
            n1077 = Less?(x=w1666, y=0.0) -> (x < y?=w1674:bool)
            n1078 = Less?(x=w1664, y=0.0) -> (x < y?=w1675:bool)
            n1079 = Greater?(x=w1688, y=500) -> (0:w1679:bool)
            n1080 = Subtract(x=w1696, y=w1687) -> (x-y=w1695:u32)
            n1081 = Or(x=w1679, y=w1680) -> (x .or. y?=w1678:bool)
            n1082 = To Double Precision Float(number=w1695) -> (double precision float=w1694:dbl)
            n1083 = And(x=w1662, y=w1671) -> (x .and. y?=w1676:bool)
            n1084 = And(x=w1674, y=w1675) -> (x .and. y?=w1677:bool)
            n1085 = local read "Å]Vx1"() -> (w1683:i32)
            n1086 = Or(x=w1676, y=w1677) -> (x .or. y?=w1663:bool)
            n1087 = Divide(x=w1694, y=1000.0) -> (x/y=w1692:dbl)
            n1088 = local read "Å]XÄ²1"() -> (w1690:i32)
            n1089 = case shown="True" w1663 {
              frame False {
              }
              frame True {
                w1697 = 200 ("x觸及位置")
                n1090 = local write "Å]XÄ²1"(w1697) -> ()
                n1091 = Wait (ms)(milliseconds to wait=u32 100) -> ()  [unwired: 1 out]
                n1092 = property on="魔王1" class="Bool (strict)"("Left"=w1697) -> ()  [unwired: 2 in, 2 out]
              }
            }
            n1093 = Multiply(x=w1692, y=w1683) -> (x*y=w1691:dbl)
            n1094 = Add(x=w1691, y=w1690) -> (x+y=w1686:dbl)
            n1095 = case shown="True" w1678 {
              tunnel: [enum16{"speed"}."speed" ("Enum") enum16{"speed"}."speed" ("Enum")] -> w1684
              tunnel: [w1699 w1706] -> w1685
              tunnel: w1687 -> [w1699 _]
              tunnel: w1686 -> [_ w1702]
              tunnel: w1683 -> [_ w1704]
              frame False {
              }
              frame True {
                n1096 = Multiply(x=w1704, y=-1.0) -> (x*y=w1701:dbl)
                n1097 = local write "Å]XÄ²1"(w1702) -> ()
                n1098 = Wait (ms)(milliseconds to wait=u32 25) -> ()  [unwired: 1 out]
                n1099 = local write "Å]Vx1"(w1701) -> ()
                n1100 = Tick Count (ms)() -> (millisecond timer value=w1706:u32)
              }
            }
            n1101 = property on="魔王1" class="Bool (strict)"("Left"=w1686) -> ()  [unwired: 2 in, 2 out]
            n1102 = Wait (ms)(milliseconds to wait=u32 10) -> ()  [unwired: 1 out]
            n1103 = property on="魔王1" class="Bool (strict)"() -> ("Left"=w1668:i32)  [unwired: 2 in, 2 out]
          }
        }
        n1104 = case shown="\"speed\"" w1518 {
          tunnel: w1519 -> [w1985]
          tunnel: [w1983] -> w1517
          tunnel: [w1982] -> w1516
          tunnel: [w1966] -> w1507
          tunnel: w1506 -> [w1965]
          tunnel: w1506 -> [w1964]
          tunnel: w1505 -> [w1963]
          tunnel: w1505 -> [w1962]
          frame "speed" {
            n1105 = Tick Count (ms)() -> (millisecond timer value=w1994:u32)
            n1106 = Greater?(x=w1965, y=400.0) -> (0:w1960:bool)
            n1107 = Greater?(x=w1963, y=400.0) -> (0:w1969:bool)
            n1108 = Less?(x=w1964, y=0.0) -> (x < y?=w1972:bool)
            n1109 = Less?(x=w1962, y=0.0) -> (x < y?=w1973:bool)
            n1110 = property on="Y障礙" class="Bool (strict)"() -> ("Top"=w1986:i32)  [unwired: 2 in, 2 out]
            n1111 = property on="Y障礙" class="Bool (strict)"() -> ("Top"=w1980:i32)  [unwired: 2 in, 2 out]
            n1112 = Less?(x=w1980, y=0) -> (x < y?=w1978:bool)
            n1113 = Greater?(x=w1986, y=400) -> (0:w1977:bool)
            n1114 = Subtract(x=w1994, y=w1985) -> (x-y=w1993:u32)
            n1115 = Or(x=w1977, y=w1978) -> (x .or. y?=w1976:bool)
            n1116 = And(x=w1960, y=w1969) -> (x .and. y?=w1974:bool)
            n1117 = And(x=w1972, y=w1973) -> (x .and. y?=w1975:bool)
            n1118 = To Double Precision Float(number=w1993) -> (double precision float=w1992:dbl)
            n1119 = Or(x=w1974, y=w1975) -> (x .or. y?=w1961:bool)
            n1120 = local read "Vy"() -> (w1981:i32)
            n1121 = local read "y觸及位置"() -> (w1988:i32)
            n1122 = Divide(x=w1992, y=1000.0) -> (x/y=w1990:dbl)
            n1123 = case shown="True" w1961 {
              frame False {
              }
              frame True {
                w1995 = 200 ("y觸及位置")
                n1124 = local write "y觸及位置"(w1995) -> ()
                n1125 = Wait (ms)(milliseconds to wait=u32 100) -> ()  [unwired: 1 out]
                n1126 = property on="Y障礙" class="Bool (strict)"("Top"=w1995) -> ()  [unwired: 2 in, 2 out]
              }
            }
            n1127 = Multiply(x=w1990, y=w1981) -> (x*y=w1989:dbl)
            n1128 = Add(x=w1989, y=w1988) -> (x+y=w1984:dbl)
            n1129 = case shown="True" w1976 {
              tunnel: [enum16{"speed"}."speed" ("Enum") enum16{"speed"}."speed" ("Enum")] -> w1982
              tunnel: [w1997 w2004] -> w1983
              tunnel: w1985 -> [w1997 _]
              tunnel: w1984 -> [_ w2000]
              tunnel: w1981 -> [_ w2002]
              frame False {
              }
              frame True {
                n1130 = local write "y觸及位置"(w2000) -> ()
                n1131 = Multiply(x=w2002, y=-1.0) -> (x*y=w1999:dbl)
                n1132 = Wait (ms)(milliseconds to wait=u32 25) -> ()  [unwired: 1 out]
                n1133 = Tick Count (ms)() -> (millisecond timer value=w2004:u32)
                n1134 = local write "Vy"(w1999) -> ()
              }
            }
            n1135 = property on="Y障礙" class="Bool (strict)"("Top"=w1984) -> ()  [unwired: 2 in, 2 out]
            n1136 = property on="Y障礙" class="Bool (strict)"() -> ("Top"=w1966:i32)  [unwired: 2 in, 2 out]
            n1137 = Wait (ms)(milliseconds to wait=u32 10) -> ()  [unwired: 1 out]
          }
        }
        n1138 = call-poly <vilib>:"Acquire Input Data.vi"("device ID"=w1515, "error in (no error)"=w1514) -> ("device ID"=w1487:refnum<k1>, "keys pressed"=w1513:T1, "error out"=w1486:errorcluster)  [unwired: 15 in]
        n1139 = Increment(x=w1467) -> (x+1=w1468:i32)
        n1140 = local write "遊玩時間"(w1468) -> ()
        n1141 = Array To Cluster(array=w1513) -> (cluster=w1504:T2)
        n1142 = Unbundle(w1504) -> ("keys pressed[0]"=w1512:T3)  [unwired: 8 out]
        n1143 = case shown="\"A\"" w1512 {
          frame Default {
          }
          frame "A" {
            n1144 = local read "X"() -> (w1957:dbl)
            n1145 = Wait (ms)(milliseconds to wait=u32 10) -> ()  [unwired: 1 out]
            n1146 = Add(x=-2.0, y=w1957) -> (x+y=w1955:dbl)
            n1147 = local write "X"(w1955) -> ()
            n1148 = property on="小精靈" class="Bool (strict)"("Left"=w1955) -> ()  [unwired: 2 in, 2 out]
          }
        }
        n1149 = case shown="\"D\"" w1512 {
          frame Default {
          }
          frame "D" {
            n1150 = local read "X"() -> (w1953:dbl)
            n1151 = Wait (ms)(milliseconds to wait=u32 10) -> ()  [unwired: 1 out]
            n1152 = Add(x=2.0, y=w1953) -> (x+y=w1951:dbl)
            n1153 = local write "X"(w1951) -> ()
            n1154 = property on="小精靈" class="Bool (strict)"("Left"=w1951) -> ()  [unwired: 2 in, 2 out]
          }
        }
        n1155 = property on="Y障礙" class="Bool (strict)"() -> ("Top"=w1488:i32)  [unwired: 2 in, 2 out]
        n1156 = property on="Y障礙" class="Bool (strict)"() -> ("Top"=w1494:i32)  [unwired: 2 in, 2 out]
        n1157 = property on="Y障礙" class="Bool (strict)"() -> ("Left"=w1501:i32)  [unwired: 2 in, 2 out]
        n1158 = property on="Y障礙" class="Bool (strict)"() -> ("Left"=w1499:i32)  [unwired: 2 in, 2 out]
        n1159 = case shown="\"W\"" w1512 {
          frame Default {
          }
          frame "W" {
            n1160 = local read "Y"() -> (w1949:dbl)
            n1161 = Wait (ms)(milliseconds to wait=u32 10) -> ()  [unwired: 1 out]
            n1162 = Add(x=-2.0, y=w1949) -> (x+y=w1947:dbl)
            n1163 = local write "Y"(w1947) -> ()
            n1164 = property on="小精靈" class="Bool (strict)"("Top"=w1947) -> ()  [unwired: 2 in, 2 out]
          }
        }
        n1165 = case shown="\"S\"" w1512 {
          frame Default {
          }
          frame "S" {
            n1166 = local read "Y"() -> (w1945:dbl)
            n1167 = Wait (ms)(milliseconds to wait=u32 10) -> ()  [unwired: 1 out]
            n1168 = Add(x=2.0, y=w1945) -> (x+y=w1943:dbl)
            n1169 = local write "Y"(w1943) -> ()
            n1170 = property on="小精靈" class="Bool (strict)"("Top"=w1943) -> ()  [unwired: 2 in, 2 out]
          }
        }
        n1171 = local read "Y"() -> (w1502:dbl)
        n1172 = local read "X"() -> (w1503:dbl)
        n1173 = Add(x=w1501, y=17) -> (x+y=w1496:i32)
        n1174 = Subtract(x=w1499, y=17) -> (x-y=w1497:i32)
        n1175 = Subtract(x=w1494, y=15) -> (x-y=w1493:i32)
        n1176 = Add(x=w1488, y=20) -> (x+y=w1489:i32)
        n1177 = In Range and Coerce(upper limit=w1496, x=w1503, lower limit=w1497) -> (In Range?=w1492:bool)  [unwired: 1 out]
        n1178 = In Range and Coerce(upper limit=w1489, x=w1502, lower limit=w1493) -> (In Range?=w1491:bool)  [unwired: 1 out]
        n1179 = And(x=w1492, y=w1491) -> (x .and. y?=w1426:bool)
        n1180 = property on="X障礙" class="Bool (strict)"() -> ("Top"=w1485:i32)  [unwired: 2 in, 2 out]
        n1181 = property on="X障礙" class="Bool (strict)"() -> ("Top"=w1479:i32)  [unwired: 2 in, 2 out]
        n1182 = property on="X障礙" class="Bool (strict)"() -> ("Left"=w1472:i32)  [unwired: 2 in, 2 out]
        n1183 = property on="X障礙" class="Bool (strict)"() -> ("Left"=w1474:i32)  [unwired: 2 in, 2 out]
        n1184 = local read "Y"() -> (w1471:dbl)
        n1185 = property on="魔王" class="Bool (strict)"() -> ("Top"=w1432:i32)  [unwired: 2 in, 2 out]
        n1186 = property on="魔王" class="Bool (strict)"() -> ("Top"=w1438:i32)  [unwired: 2 in, 2 out]
        n1187 = property on="魔王" class="Bool (strict)"() -> ("Left"=w1445:i32)  [unwired: 2 in, 2 out]
        n1188 = property on="魔王" class="Bool (strict)"() -> ("Left"=w1443:i32)  [unwired: 2 in, 2 out]
        n1189 = local read "X"() -> (w1470:dbl)
        n1190 = local read "Y"() -> (w1446:dbl)
        n1191 = local read "X"() -> (w1447:dbl)
        n1192 = property on="X障礙 2" class="Bool (strict)"() -> ("Top"=w1398:i32)  [unwired: 2 in, 2 out]
        n1193 = property on="X障礙 2" class="Bool (strict)"() -> ("Top"=w1392:i32)  [unwired: 2 in, 2 out]
        n1194 = property on="X障礙 2" class="Bool (strict)"() -> ("Left"=w1385:i32)  [unwired: 2 in, 2 out]
        n1195 = property on="X障礙 2" class="Bool (strict)"() -> ("Left"=w1387:i32)  [unwired: 2 in, 2 out]
        n1196 = property on="魔王2" class="Bool (strict)"() -> ("Top"=w1302:i32)  [unwired: 2 in, 2 out]
        n1197 = property on="魔王2" class="Bool (strict)"() -> ("Top"=w1308:i32)  [unwired: 2 in, 2 out]
        n1198 = property on="Y障礙 2" class="Bool (strict)"() -> ("Top"=w1367:i32)  [unwired: 2 in, 2 out]
        n1199 = property on="Y障礙 2" class="Bool (strict)"() -> ("Top"=w1373:i32)  [unwired: 2 in, 2 out]
        n1200 = property on="魔王2" class="Bool (strict)"() -> ("Left"=w1315:i32)  [unwired: 2 in, 2 out]
        n1201 = property on="魔王2" class="Bool (strict)"() -> ("Left"=w1313:i32)  [unwired: 2 in, 2 out]
        n1202 = property on="Y障礙 2" class="Bool (strict)"() -> ("Left"=w1380:i32)  [unwired: 2 in, 2 out]
        n1203 = property on="Y障礙 2" class="Bool (strict)"() -> ("Left"=w1378:i32)  [unwired: 2 in, 2 out]
        n1204 = property on="魔王1" class="Bool (strict)"() -> ("Top"=w1348:i32)  [unwired: 2 in, 2 out]
        n1205 = property on="魔王1" class="Bool (strict)"() -> ("Top"=w1342:i32)  [unwired: 2 in, 2 out]
        n1206 = property on="魔王1" class="Bool (strict)"() -> ("Left"=w1335:i32)  [unwired: 2 in, 2 out]
        n1207 = property on="魔王1" class="Bool (strict)"() -> ("Left"=w1337:i32)  [unwired: 2 in, 2 out]
        n1208 = local read "X"() -> (w1466:dbl)
        n1209 = local read "Y"() -> (w1465:dbl)
        n1210 = Add(x=w1472, y=17) -> (x+y=w1477:i32)
        n1211 = Subtract(x=w1474, y=17) -> (x-y=w1476:i32)
        n1212 = Subtract(x=w1479, y=15) -> (x-y=w1480:i32)
        n1213 = Add(x=w1485, y=20) -> (x+y=w1484:i32)
        n1214 = local read "Y"() -> (w1384:dbl)
        n1215 = local read "Y"() -> (w1316:dbl)
        n1216 = local read "Y"() -> (w1381:dbl)
        n1217 = local read "Y"() -> (w1334:dbl)
        n1218 = local read "X"() -> (w1383:dbl)
        n1219 = local read "X"() -> (w1317:dbl)
        n1220 = local read "X"() -> (w1382:dbl)
        n1221 = local read "X"() -> (w1333:dbl)
        n1222 = Add(x=w1445, y=17) -> (x+y=w1440:i32)
        n1223 = Subtract(x=w1443, y=17) -> (x-y=w1441:i32)
        n1224 = Subtract(x=w1438, y=15) -> (x-y=w1437:i32)
        n1225 = Add(x=w1432, y=20) -> (x+y=w1433:i32)
        n1226 = In Range and Coerce(upper limit=w1477, x=w1470, lower limit=w1476) -> (In Range?=w1481:bool)  [unwired: 1 out]
        n1227 = In Range and Coerce(upper limit=w1484, x=w1471, lower limit=w1480) -> (In Range?=w1482:bool)  [unwired: 1 out]
        n1228 = In Range and Coerce(upper limit=40.0, x=w1466, lower limit=-20.0) -> (In Range?=w1464:bool)  [unwired: 1 out]
        n1229 = In Range and Coerce(upper limit=25.0, x=w1465, lower limit=-18.0) -> (In Range?=w1463:bool)  [unwired: 1 out]
        n1230 = Add(x=w1385, y=17) -> (x+y=w1390:i32)
        n1231 = Subtract(x=w1387, y=17) -> (x-y=w1389:i32)
        n1232 = Subtract(x=w1392, y=15) -> (x-y=w1393:i32)
        n1233 = Add(x=w1315, y=17) -> (x+y=w1310:i32)
        n1234 = Add(x=w1380, y=17) -> (x+y=w1375:i32)
        n1235 = Subtract(x=w1313, y=17) -> (x-y=w1311:i32)
        n1236 = Subtract(x=w1308, y=15) -> (x-y=w1307:i32)
        n1237 = Subtract(x=w1378, y=17) -> (x-y=w1376:i32)
        n1238 = Subtract(x=w1373, y=15) -> (x-y=w1372:i32)
        n1239 = Add(x=w1335, y=17) -> (x+y=w1340:i32)
        n1240 = Subtract(x=w1337, y=17) -> (x-y=w1339:i32)
        n1241 = Subtract(x=w1342, y=15) -> (x-y=w1343:i32)
        n1242 = Add(x=w1398, y=20) -> (x+y=w1397:i32)
        n1243 = Add(x=w1302, y=20) -> (x+y=w1303:i32)
        n1244 = Add(x=w1367, y=20) -> (x+y=w1368:i32)
        n1245 = Add(x=w1348, y=20) -> (x+y=w1347:i32)
        n1246 = In Range and Coerce(upper limit=w1440, x=w1447, lower limit=w1441) -> (In Range?=w1436:bool)  [unwired: 1 out]
        n1247 = In Range and Coerce(upper limit=w1433, x=w1446, lower limit=w1437) -> (In Range?=w1435:bool)  [unwired: 1 out]
        n1248 = And(x=w1481, y=w1482) -> (x .and. y?=w1425:bool)
        n1249 = And(x=w1464, y=w1463) -> (x .and. y?=w1423:bool)
        n1250 = In Range and Coerce(upper limit=w1390, x=w1383, lower limit=w1389) -> (In Range?=w1394:bool)  [unwired: 1 out]
        n1251 = In Range and Coerce(upper limit=w1397, x=w1384, lower limit=w1393) -> (In Range?=w1395:bool)  [unwired: 1 out]
        n1252 = In Range and Coerce(upper limit=w1310, x=w1317, lower limit=w1311) -> (In Range?=w1306:bool)  [unwired: 1 out]
        n1253 = In Range and Coerce(upper limit=w1303, x=w1316, lower limit=w1307) -> (In Range?=w1305:bool)  [unwired: 1 out]
        n1254 = In Range and Coerce(upper limit=w1375, x=w1382, lower limit=w1376) -> (In Range?=w1371:bool)  [unwired: 1 out]
        n1255 = In Range and Coerce(upper limit=w1368, x=w1381, lower limit=w1372) -> (In Range?=w1370:bool)  [unwired: 1 out]
        n1256 = In Range and Coerce(upper limit=w1340, x=w1333, lower limit=w1339) -> (In Range?=w1344:bool)  [unwired: 1 out]
        n1257 = In Range and Coerce(upper limit=w1347, x=w1334, lower limit=w1343) -> (In Range?=w1345:bool)  [unwired: 1 out]
        n1258 = And(x=w1436, y=w1435) -> (x .and. y?=w1424:bool)
        n1259 = And(x=w1394, y=w1395) -> (x .and. y?=w1366:bool)
        n1260 = And(x=w1306, y=w1305) -> (x .and. y?=w1301:bool)
        n1261 = And(x=w1371, y=w1370) -> (x .and. y?=w1365:bool)
        n1262 = And(x=w1344, y=w1345) -> (x .and. y?=w1332:bool)
        n1263 = Compound Arithmetic op=OR(w1301, w1332, w1363, w1364, w1365, w1366, w1413, w1414, w1415, w1416, w1423, w1431, w1430, w1429, w1428, w1427, w1426, w1425, w1424) -> (w1469:bool)
      }
      n1264 = call-poly <vilib>:"Close Input Device.vi"("error in (no error)"=w1292, "device ID"=w1293) -> ()  [unwired: 8 in, 1 out]
      n1265 = case shown="True" w1281 {
        frame False {
          n1266 = One Button Dialog(message="就跟你說 Crazy 還玩?", button name ("OK")="иゆM") -> ()  [unwired: 1 out]
        }
        frame True {
          n1267 = One Button Dialog(message="你太閒了....", button name ("OK")=".....") -> ()  [unwired: 1 out]
        }
      }
    }
  }
  "終點" <- TRUE ("Boolean 3")
